vi "STED Control V5.vi"() -> ()   [LabVIEW 2014]
uses:
  Type Defs/Image Acquisition Parameters.ctl
  Laser Controls.ctl
  Detectors.ctl
  Stage Control.ctl
  Focus Control.ctl
  Tools VIs/GrpahTools.ctl
  FPGA-7842R-Reference.ctl
  Scan Parameters.ctl
  Manual Controls V2.ctl
  <vilib>/Utility/miscctls.llb/LVPositionTypeDef.ctl
  <vilib>/Utility/miscctls.llb/LVRectTypeDef.ctl
  Controls/StageStates.ctl
panel:
  in  "Cursor":bool
  in  "Graph Mode":T1(radio)=enum."FullChip"
  in  "Colormap":T2(ring)
  in  "Active Channel":u16(ring) items=["Channel 1"]
  in  "Graph Tools":T3
  in  "Tab Control":T4(tab)
  in  "SLM":bool
  in  "DM":bool
  in  "Timing":bool
  in  "Pixelfly":bool
  in  "Focus Control":T5
  in  "Stage Control":T6={"Halt"=FALSE, "Home"=FALSE, "Down Stage"=FALSE, "Right Stage"=FALSE, "Up Stage"=FALSE, "Left Stage"=FALSE, "X Position"=1.0, "Y Position"=1.0, "Step Size (um)"=enum."1", "Velocity"=enum."Low"} {"Y Position" min=1.0 max=24.0; "X Position" min=1.0 max=24.0}
  out "Channel 6":sgl[][](graph)
  out "Channel 5":sgl[][](graph)
  out "Channel 4":sgl[][](graph)
  out "Channel 3":sgl[][](graph)
  out "Channel 2":sgl[][](graph)
  in  "Detectors":T7
  in  "Laser Controls":T8 {"590 Power (V)" scale=0.0..3.0; "STED Power (V)" scale=0.0..10.0}
  in  "Save File Path":path
  in  "Capture":bool
  out "Channel 1":sgl[][](graph)
  in  "Image Acquisition Parameters":T9={"Scan Type"=enum."Beam Scanning", "Scan Mode"=enum."XY", "Fast Axis Frequency (Hz)"=16110.0, "Image Format"=256, "Line Accumulations"=100, "Frames Per Capture"=1, "Frames Accumulations"=1, "Image Dimension (um)"=[15.0, 15.0], "Number of Z Steps"=1, "Z Steps Size (um)"=1.0, "Pixel Size (nm)"=[58.59375, 58.59375]} {"Z Steps Size (um)" min=0.0; "Number of Z Steps" min=1; "Frames Accumulations" min=1; "Frames Per Capture" min=1; "Line Accumulations" min=1; "Image Format" items=["64 x 64"=64, "128 x 128"=128, "256 x 256"=256, "512 x 512"=512, "1024 x 1024"=1024, "2048 x 2048"=2048]}
  in  "Live":bool
  in  "Exit":bool
  # "XY"
  # "Z"
  # "Length"
  # "Height"
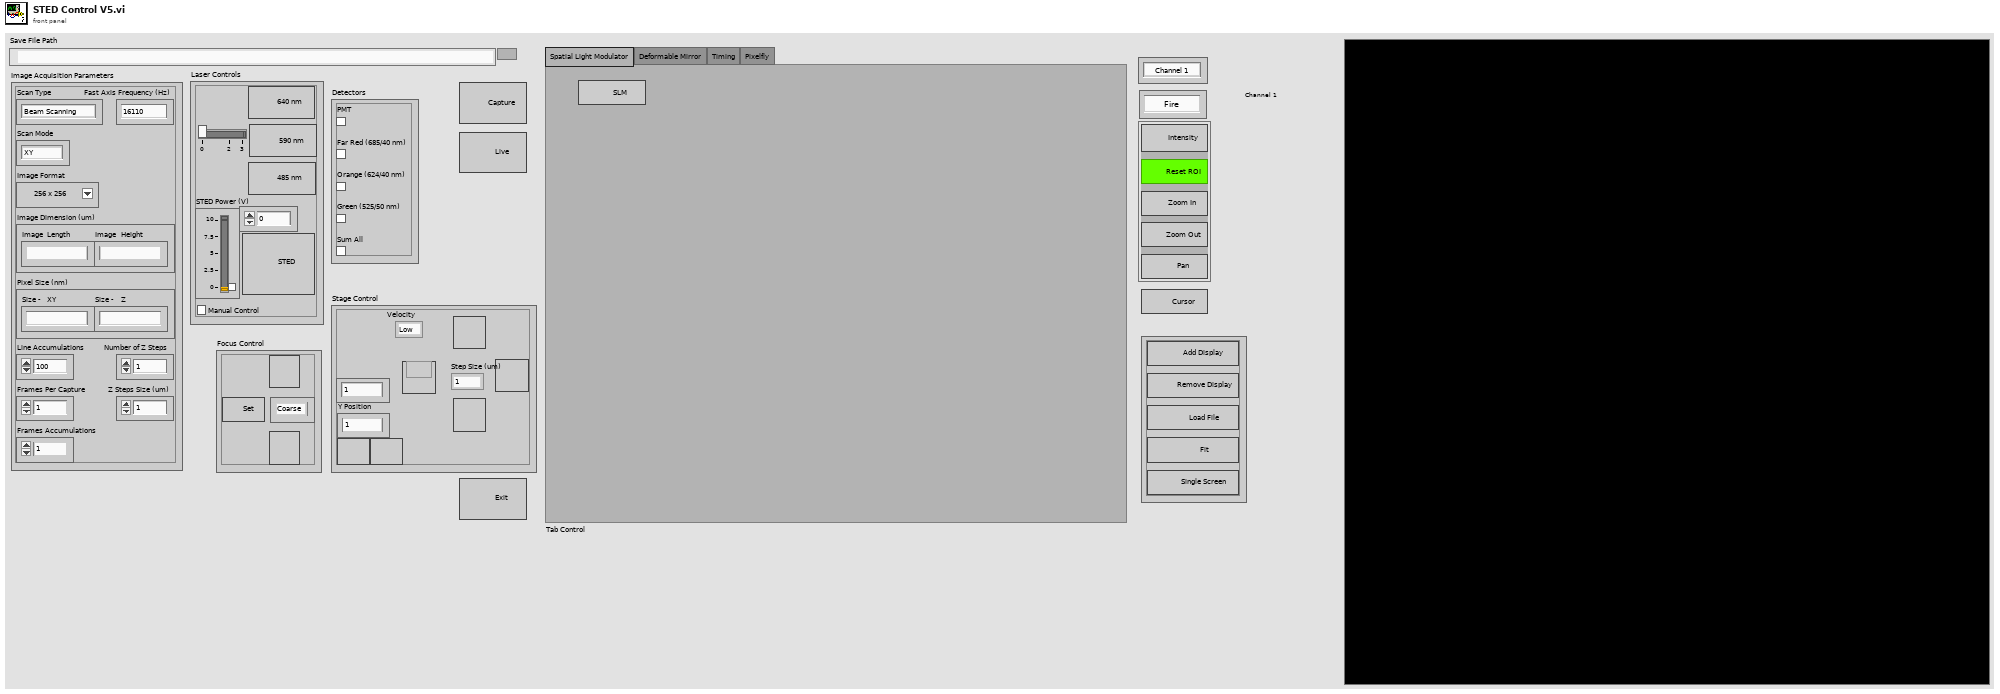
[diagram p1: front panel]
types:
  T1 = enum32{"GetIntensity", "FullChip", "ZoomIn", "ZoomOut", "Pan"}
  T2 = enum16{"Fire", "Gray", "Red", "Green", "Blue", "Cyan", "Magenta", "Yellow", "Red-White", "Green-White", "Blue-White", "Glow"}
  T3 = typedef "GrpahTools.ctl" = cluster{"Add Display":bool, "Remove Display":bool, "Single Screen":bool, "Load File":bool, "Fit":bool}
  T4 = enum32{"Spatial Light Modulator", "Deformable Mirror", "Timing", "Pixelfly"}
  T5 = typedef "Focus Control.ctl" = cluster{"ZoomUp":bool, "ZoomDown":bool, "ZoomStepI16":enum16{"Coarse", "Medium", "Fine"}, "SetZoom":bool}
  T6 = typedef "Stage Control.ctl" = cluster{"Halt":bool, "Home":bool, "Down Stage":bool, "Right Stage":bool, "Up Stage":bool, "Left Stage":bool, "X Position":dbl, "Y Position":dbl, "Step Size (um)":enum16{"1", "2", "5", "10", "15", "20", "50", "100", "500"}, "Velocity":enum16{"Low", "Medium", "High"}}
  T7 = typedef "Detectors.ctl" = cluster{"PMT":bool, "Far Red (685/40 nm)":bool, "Orange (624/40 nm)":bool, "Green (525/50 nm)":bool, "Sum All":bool}
  T8 = typedef "Laser Controls.ctl" = cluster{"STED Power (V)":dbl, "590 Power (V)":dbl, "STED":bool, "640 nm":bool, "590 nm":bool, "485 nm":bool, "Manual Control":bool}
  T9 = typedef "Image Acquisition Parameters.ctl" = cluster{"Scan Type":enum16{"Sample Scanning", "Beam Scanning"}, "Scan Mode":enum16{"XY", "XZ", "YZ", "XYZ"}, "Fast Axis Frequency (Hz)":dbl, "Image Format":u16, "Line Accumulations":u16, "Frames Per Capture":u16, "Frames Accumulations":u16, "Image Dimension (um)":dbl[], "Number of Z Steps":u8, "Z Steps Size (um)":dbl, "Pixel Size (nm)":dbl[]}
  T10 = typedef "Manual Controls V2.ctl" = cluster{"Galvo 1 Position (I16)":i16, "Galvo 2 Position (I16)":i16, "X Axis Voltage (I16)":i16, "Y Axis Voltage (I16)":i16, "Z Axis Voltage (I16)":i16, "Res Mirror Amp (I16)":i16, "Res Mirror Mute":bool}
  T11 = typedef "Scan Parameters.ctl" = cluster{"Fast_Ax_Amp_V":dbl, "Fast_Ax_Off_V":dbl, "Slow_Ax_Amp_V":dbl, "Slow_Ax_Off_V ":dbl, "Slow_Ax_Max_V_VperS":dbl, "Slow_Ax1_Del25ns":i32, "Slow_Ax2_Del25ns":i32, "Stage_X_Off_V":dbl, "Stage_Y_Off_V":dbl, "Stage_Z_Off_V":dbl, "Galvo1_Off_V":dbl, "Galvo2_Off_V":dbl, "Last_Scan_Mode":enum16{"XY", "XZ", "YZ", "XYZ"}, "Current_Scan_Mode":enum16{"XY", "XZ", "YZ", "XYZ"}, "Fly_Back_Lines":u16, "Linear_Ramp_End":u32, "Z_Step_I16":i16, "Z_Start_I16":i16, "Laser_States _U32":u32, "590_Voltage_I16":i16, "775_AOM_Volt_I16":i16, "Blanking OFF":bool, "Unused_Axis_I16":i16}
  T12 = typedef "FPGA-7842R-Reference.ctl" = enum16{"Stage Control", "Laser Control", "Unused Axis I16", "Exit", "Set Res Mirror", "Set Galvo", "Default", "Close FPGA", "Stop Waveforms", "Start Waveforms", "Shutter Control", "Initialize"}
  T13 = enum8{"Enabled", "Disabled", "Disabled and Grayed Out"}
  T14 = typedef "StageStates.ctl" = enum16{"POSITION", "MVR", "MOVE", "HALT", "ONTARGET", "ERROR", "EXIT", "HOME", "ZEROPOS", "NANOPOS", "QUIT", "ANALOG"}
  T15 = typedef "StageStates.ctl" = enum16{"POSITION", "MVR", "MOVE", "HALT", "ONTARGET", "ERROR", "EXIT", "HOME", "ZEROPOS", "NANOPOS", "QUIT", "SERVO", "JOYSTICK", "ANALOG"}
  T16 = typedef "LVPositionTypeDef.ctl" = cluster{"Left":i32, "Top":i32}
  T17 = typedef "LVRectTypeDef.ctl" = cluster{"Left":i16, "Top":i16, "Right":i16, "Bottom":i16}
  T18 = enum32{"Invalid", "Standard", "Closed", "Hidden", "Minimized", "Maximized"}
  T19 = cluster{"Halt":bool, "Home":bool, "Down Stage":bool, "Right Stage":bool, "Up Stage":bool, "Left Stage":bool, "X Position":bool, "Y Position":bool, "Step Size (um)":bool, "Velocity":bool}
  T20 = enum16{"1", "2", "5", "10", "15", "20", "50", "100", "500"}
  T21 = typedef "Scanning Conversions.ctl" = cluster{"Stage X Axis (Volts/um)":dbl, "Stage Y Axis (Volts/um)":dbl, "Stage Z Axis (Volts/um)":dbl}
  T22 = cluster{"Scan Type":bool, "Scan Mode":bool, "Fast Axis Frequency (Hz)":bool, "Image Format":bool, "Line Accumulations":bool, "Frames Per Capture":bool, "Frames Accumulations":bool, "Image Dimension (um)":bool[], "Number of Z Steps":bool, "Z Steps Size (um)":bool, "Pixel Size (nm)":bool[]}
  T23 = typedef "LVAllMonitorsDisplayTypeDef.ctl" = cluster{"Bounds":cluster{"Left":i16, "Top":i16, "Right":i16, "Bottom":i16}, "Depth":i16}[]
  T24 = cluster{"Bounds":cluster{"Left":i16, "Top":i16, "Right":i16, "Bottom":i16}, "Depth":i16}
  T25 = typedef "IMAQ Image.ctl" = refnum<image>
  T26 = typedef "Waveform Data.ctl" = cluster{"Waveform Scan Parameters":cluster{"Scanning Mode":u8, "Fast Axis WF Length (Elements)":i32, "Fast Axis Sample Period (Ticks)":u32, "Slow Axis 1 WF Length (Elements)":i32, "Slow Axis 1 Sample Period (Ticks)":u32, "Slow Axis 1 Delay (25 ns) Steps":i32, "Slow Axis 2 WFLength (Elements)":i32, "Slow Axis 2 Sample Period (Ticks)":u32, "Slow Axis 2 Delay (25 ns) Steps":i32}, "Fast Axis Waveform":dbl[], "Slow Axis 1 Waveform":dbl[], "Slow Axis 2 Waveform":dbl[]}
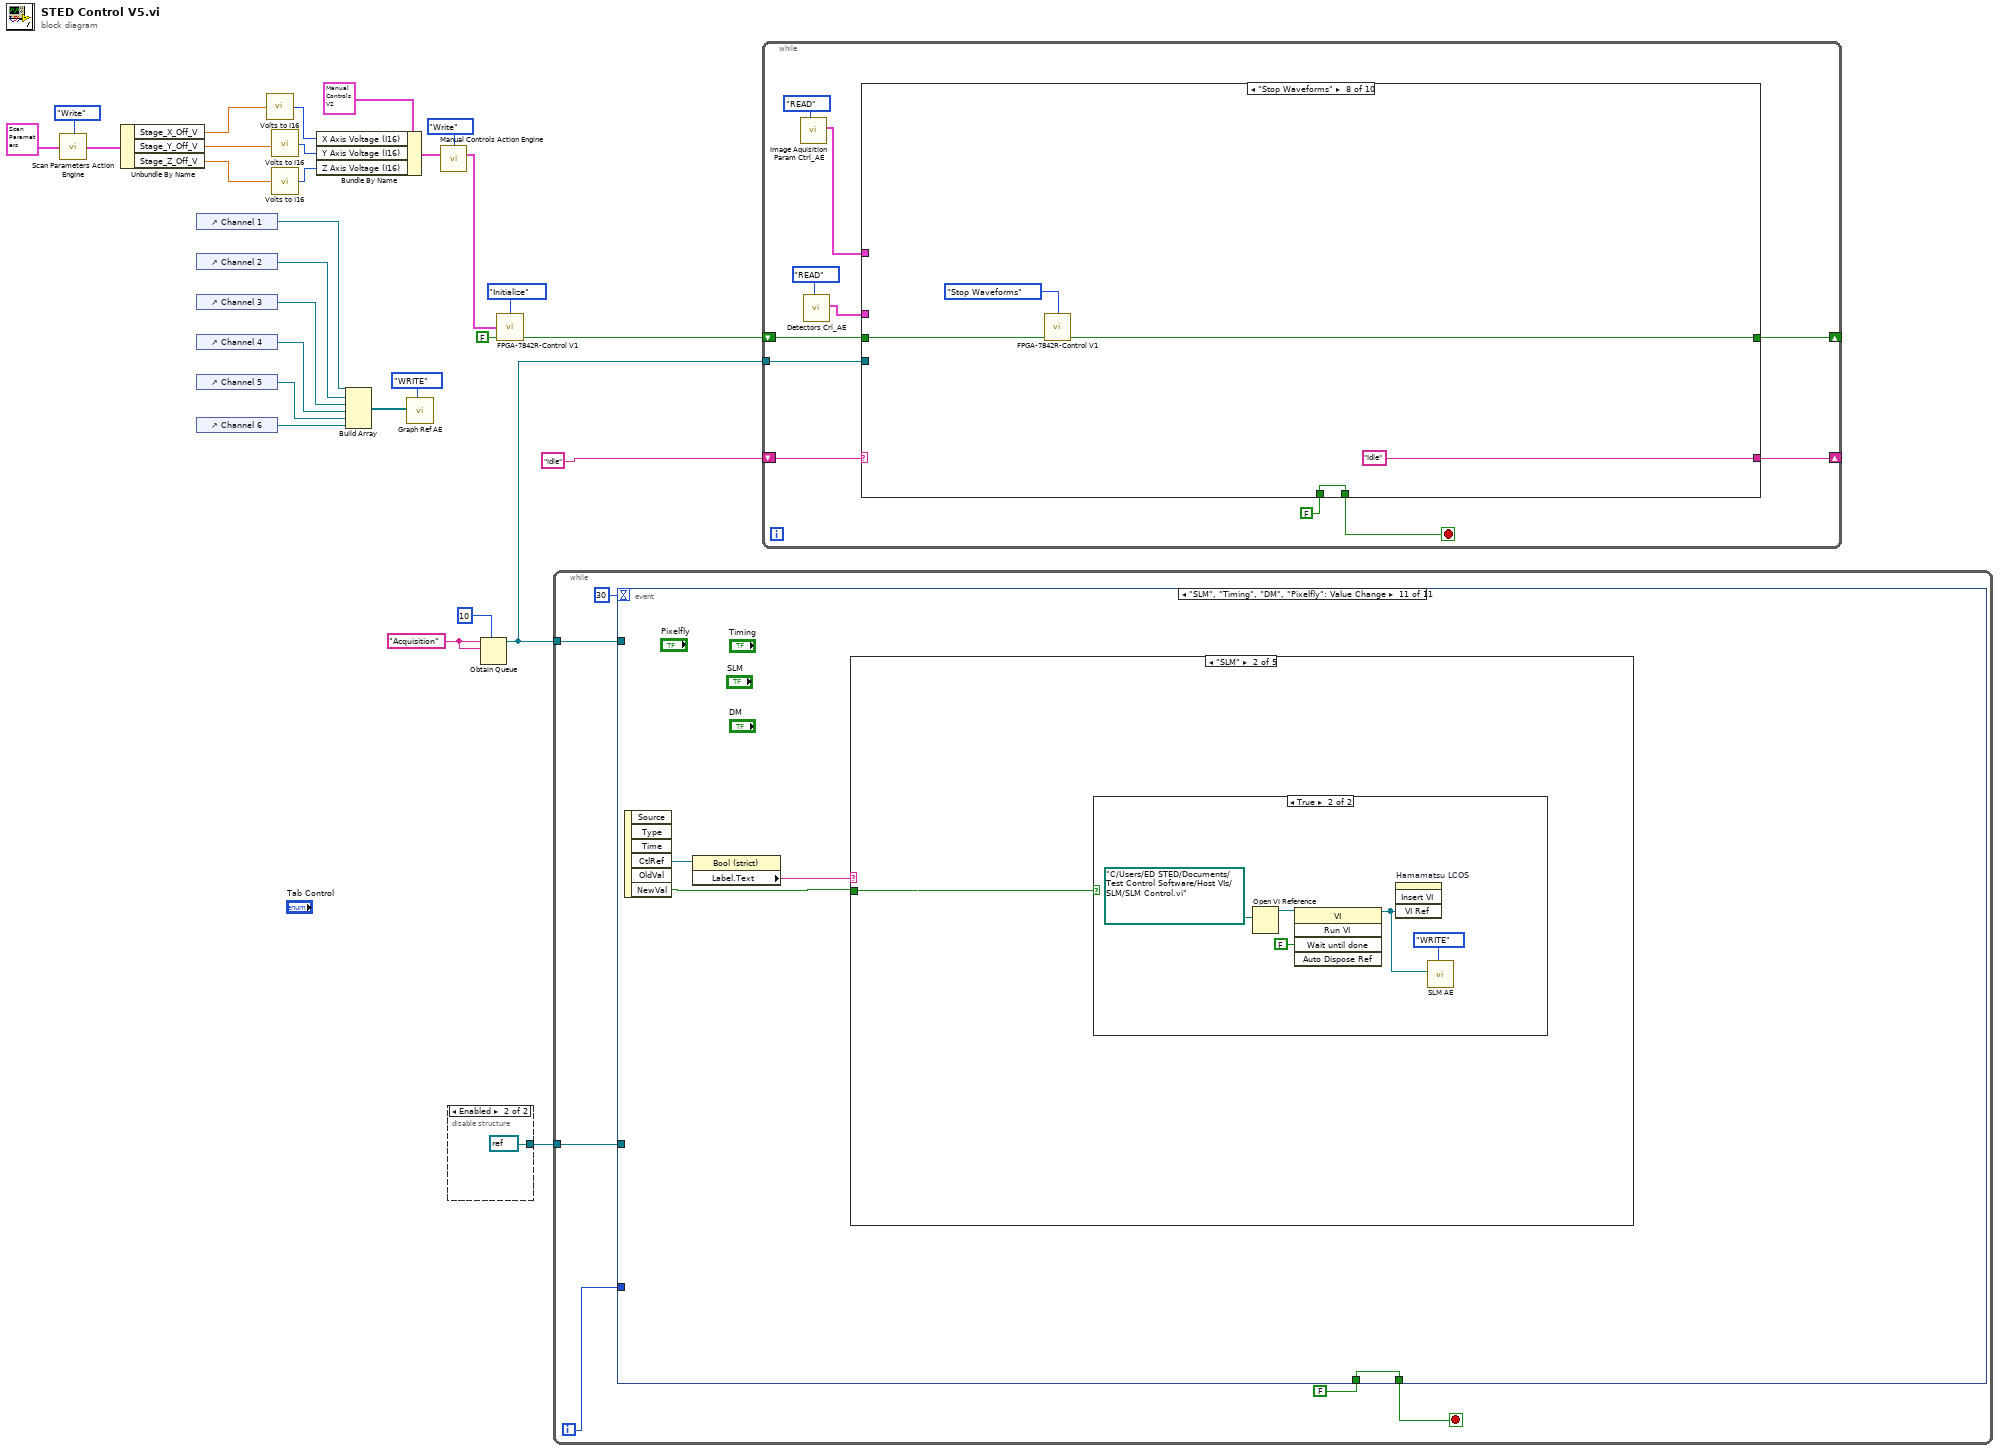
[diagram p0: block diagram]
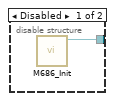
[diagram p2: hidden frame]
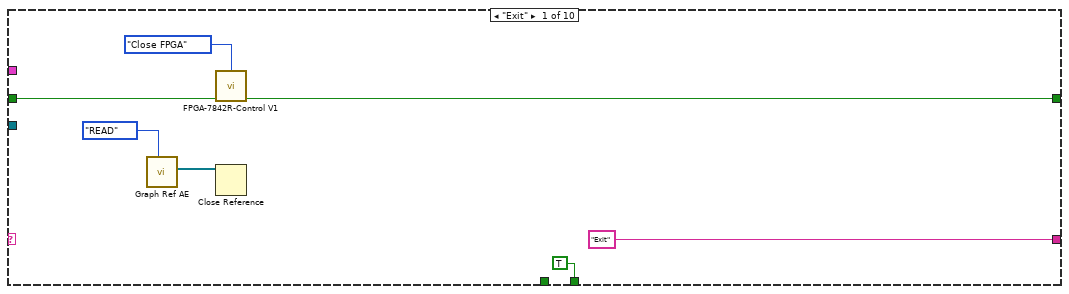
[diagram p3: hidden frame]
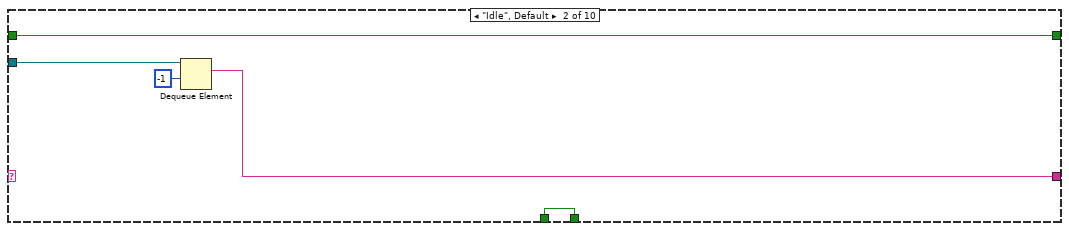
[diagram p4: hidden frame]
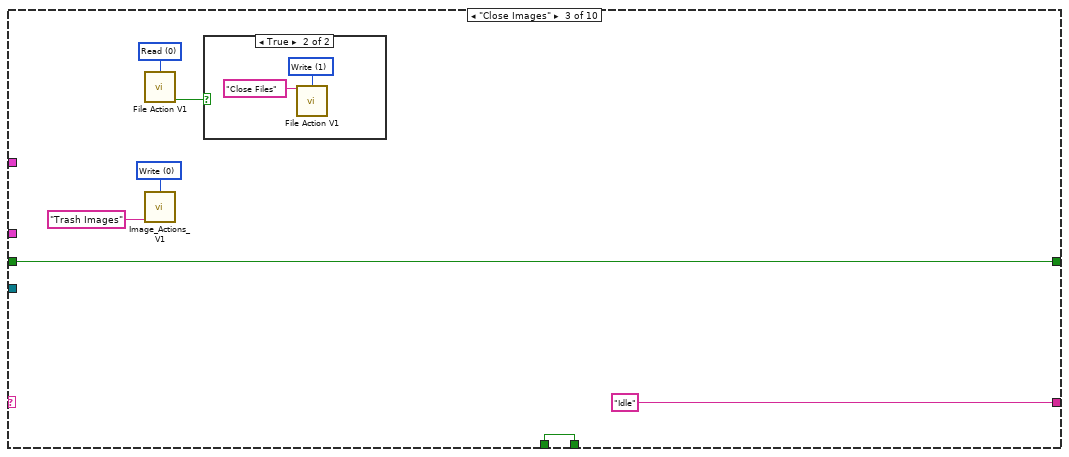
[diagram p5: hidden frame]
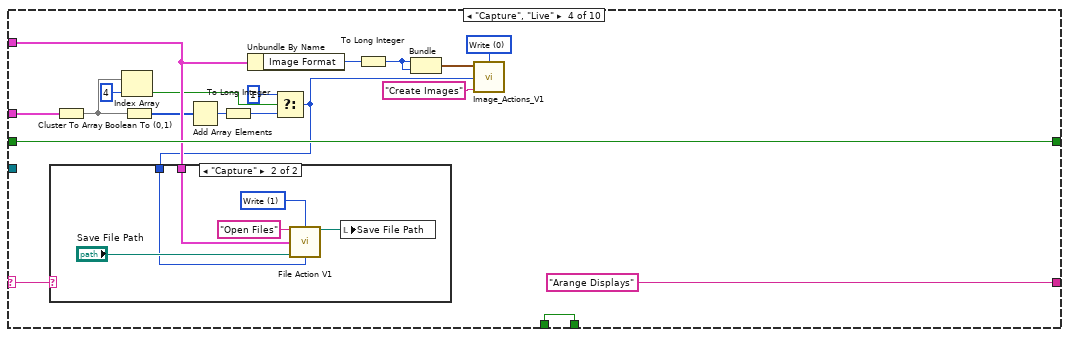
[diagram p7: hidden frame]
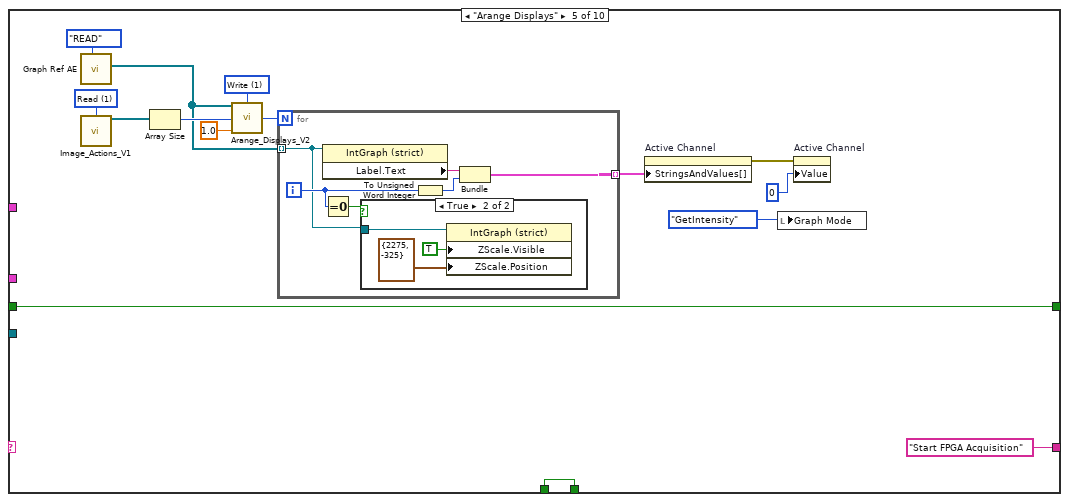
[diagram p9: hidden frame]
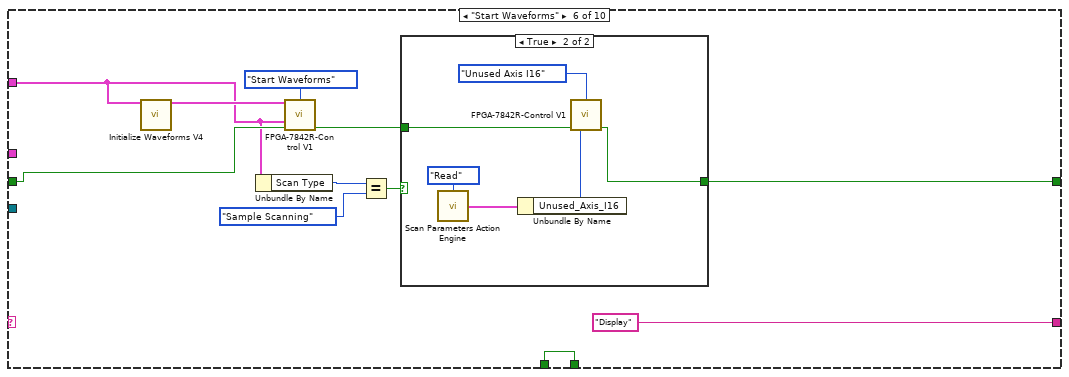
[diagram p11: hidden frame]
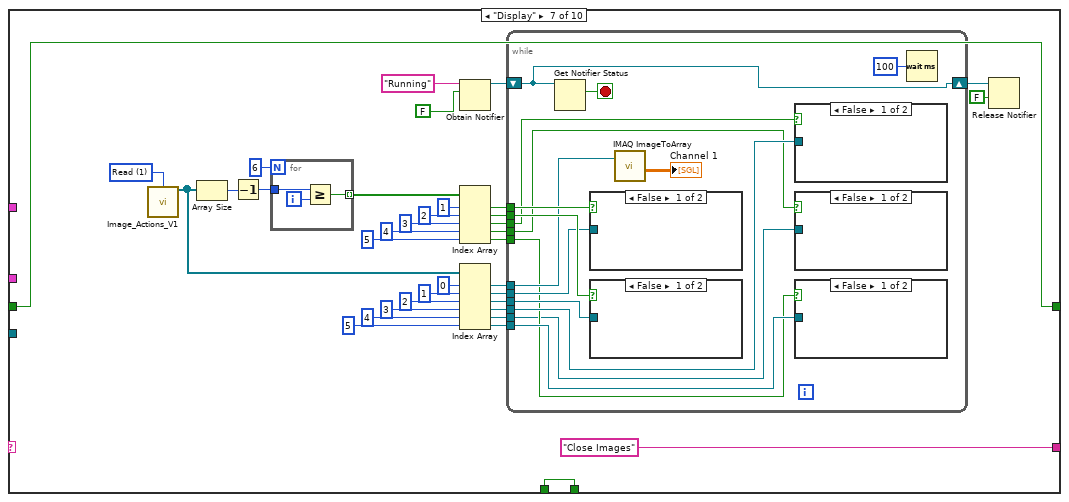
[diagram p13: hidden frame]
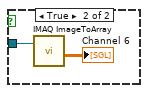
[diagram p14: hidden frame]
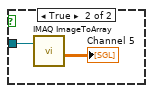
[diagram p15: hidden frame]
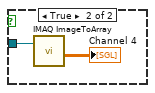
[diagram p16: hidden frame]
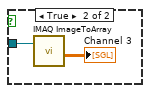
[diagram p17: hidden frame]
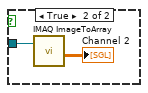
[diagram p18: hidden frame]
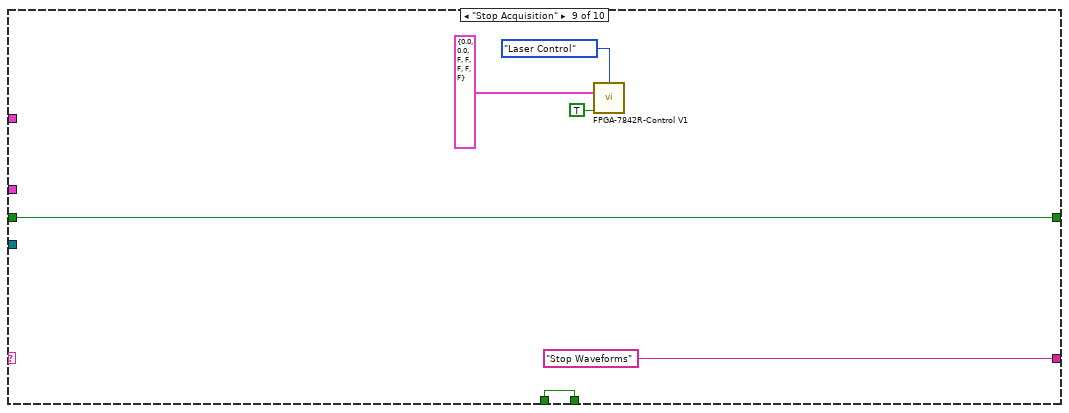
[diagram p19: hidden frame]
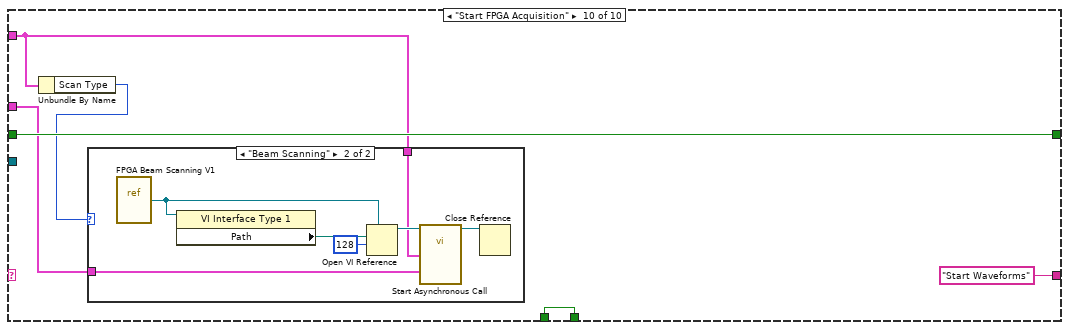
[diagram p20: hidden frame]
diagram:
  w28 = "Acquisition" ("name (unnamed)")
  n1 = call "Scan Parameters Action Engine.vi"("Action"=enum16{"Read", "Write"}."Write", "Scan Parameters IN"=T11 {"Fast_Ax_Amp_V"=0.0, "Fast_Ax_Off_V"=0.0, "Slow_Ax_Amp_V"=0.0, "Slow_Ax_Off_V "=0.0, "Slow_Ax_Max_V_VperS"=0.0, "Slow_Ax1_Del25ns"=0, "Slow_Ax2_Del25ns"=0, "Stage_X_Off_V"=5.0, "Stage_Y_Off_V"=5.0, "Stage_Z_Off_V"=5.0, "Galvo1_Off_V"=0.0, "Galvo2_Off_V"=0.0, "Last_Scan_Mode"=enum."XY", "Current_Scan_Mode"=enum."XY", "Fly_Back_Lines"=0, "Linear_Ramp_End"=0, "Z_Step_I16"=0, "Z_Start_I16"=0, "Laser_States _U32"=0, "590_Voltage_I16"=0, "775_AOM_Volt_I16"=0, "Blanking OFF"=FALSE, "Unused_Axis_I16"=16384}) -> ("Scan Parameters OUT"=w11:T11)  [unwired: 13 in]
  n2 = Unbundle By Name(w11) -> ("Stage_X_Off_V"=w7:dbl, "Stage_Y_Off_V"=w6:dbl, "Stage_Z_Off_V"=w5:dbl)
  n3 = control-ref of="Channel 1"() -> (w3:refnum<vi>)
  n4 = control-ref of="Channel 2"() -> (w20:refnum<vi>)
  n5 = control-ref of="Channel 3"() -> (w4:refnum<vi>)
  n6 = control-ref of="Channel 4"() -> (w19:refnum<vi>)
  n7 = control-ref of="Channel 5"() -> (w18:refnum<vi>)
  n8 = control-ref of="Channel 6"() -> (w17:refnum<vi>)
  n9 = call "Volts to I16.vi"("Voltage (V)"=w7) -> ("I16"=w8:i16)  [unwired: 13 in, 1 out]
  n10 = call "Volts to I16.vi"("Voltage (V)"=w6) -> ("I16"=w9:i16)  [unwired: 13 in, 1 out]
  n11 = call "Volts to I16.vi"("Voltage (V)"=w5) -> ("I16"=w10:i16)  [unwired: 13 in, 1 out]
  n12 = Bundle By Name(cluster=T10 {"Galvo 1 Position (I16)"=-280, "Galvo 2 Position (I16)"=0, "X Axis Voltage (I16)"=16384, "Y Axis Voltage (I16)"=16384, "Z Axis Voltage (I16)"=16384, "Res Mirror Amp (I16)"=0, "Res Mirror Mute"=FALSE} ("Manual Controls"), "X Axis Voltage (I16)"=w8, "Y Axis Voltage (I16)"=w9, "Z Axis Voltage (I16)"=w10) -> (w12:T10)
  n13 = Build Array(w3, w20, w4, w19, w18, w17) -> (w1:refnum<vi>[])
  n14 = call "Graph Ref AE.vi"("Action"=enum16{"READ", "WRITE"}."WRITE", "Graph Ref In"=w1) -> ()  [unwired: 9 in, 1 out]
  n15 = call "Manual Controls Action Engine.vi"("Action"=enum16{"Read", "Write"}."Write", "Manual Controls In"=w12) -> ("Manual Controls Out"=w14:T10)  [unwired: 13 in]
  n16 = disable-structure shown="Enabled" {
    disable-tunnel: [w30 refnum<visa-resource-name> refnum ("VISA Refnum out")] -> w16
    frame Disabled {
      n17 = call "M686_Init.vi"() -> ("VISA Refnum out"=w30:refnum<visa-resource-name>)  [unwired: 9 in, 2 out]
    }
    frame Enabled {
    }
  }
  n18 = Obtain Queue(max queue size (-1, unlimited)=10, name (unnamed)=w28, element data type=w28) -> (queue out=w26:refnum<queue>)  [unwired: 2 in, 2 out]
  n19 = call "FPGA-7842R-Control V1.vi"("Action"=FPGA-7842R-Reference."Initialize", "Manual Controls"=w14, "Initialize"=FALSE) -> ("Initalized"=w23:bool)  [unwired: 11 in, 1 out]
  n20 = while {
    tunnel: w26 -> [w35]
    tunnel: w16 -> [w33]
    i -> [w32]
    stop <- w37 stop-if-true
    n21 = event shown="[10] \"SLM\", \"Timing\", \"DM\", \"Pixelfly\": Value Change" {
      selector: _ -> [_ _ _ _ _ _ _ _ _ _ _]
      dyn-events: _ -> [_ _ _ _ _ _ _ _ _ _ _]
      timeout: 30 -> [_ _ _ _ _ _ _ _ _ _ _]
      tunnel: [w54 w88 w107 w117 w305 w332 w369 w408 w523 w601 w702] -> w37
      tunnel: FALSE -> [_ w88 w107 w117 w305 w332 w369 w408 w523 w601 w702]
      tunnel: w35 -> [w53 w87 w101 _ _ _ _ _ _ _ _]
      tunnel: w33 -> [w50 _ _ w116 _ _ _ _ _ _ _]
      tunnel: w32 -> [_ _ w99 _ _ _ _ _ _ _ _]
      event "Exit": Value Change {
        n22 = event-data() -> ("CtlRef"=w52:refnum<vi>, "NewVal"=w54:bool)  [unwired: 1 in, 4 out]
        n23 = disable-structure shown="Disabled" {
          disable-tunnel: w50 -> [w55 _]
          frame Disabled {
            n24 = call "M686_Quit.vi"("VISA Refnum in"=w55) -> ()  [unwired: 11 in]
          }
          frame Enabled {
          }
        }
        n25 = call "SLM AE.vi"("Action"=enum16{"READ", "WRITE"}."READ") -> ("SLM Ref Out"=w47:refnum<vi>)  [unwired: 10 in]
        n26 = Not A Number/Path/Refnum?(number/path/refnum=w47) -> (NaN/Path/Refnum?=w48:bool)
        n27 = case shown="False" w48 {
          tunnel: w47 -> [w71 _]
          frame False {
            n28 = To Variant(anything=TRUE) -> (Variant=w72:variant)
            n29 = invoke class="VI" method="Ctrl Val.Set"(reference=w71, "Control Name"="Exit", "Value"=w72) -> (reference out=w75:refnum<vi>)  [unwired: 2 in, 4 out]
            n30 = Close Reference(reference=w75) -> ()  [unwired: 1 in, 1 out]
          }
          frame True {
          }
        }
        n31 = property class="Bool"(reference=w52) -> ("Label.Text"=w51:string)  [unwired: 1 in, 2 out]
        n32 = Enqueue Element(queue=w53, element=w51) -> ()  [unwired: 2 in, 3 out]
        n33 = call "GateDelay AE.vi"("Action"=enum16{"READ", "WRITE"}."READ") -> ("Gate Delay Ref Out"=w46:refnum<vi>)  [unwired: 10 in]
        n34 = call "DM_Ref_AE.vi"("Action"=enum16{"READ", "WRITE"}."READ") -> ("DM Ref Out"=w41:refnum<vi>)  [unwired: 10 in]
        n35 = Not A Number/Path/Refnum?(number/path/refnum=w46) -> (NaN/Path/Refnum?=w45:bool)
        n36 = case shown="False" w45 {
          tunnel: w46 -> [w66 _]
          frame False {
            n37 = To Variant(anything=TRUE) -> (Variant=w67:variant)
            n38 = invoke class="VI" method="Ctrl Val.Set"(reference=w66, "Control Name"="Exit", "Value"=w67) -> (reference out=w70:refnum<vi>)  [unwired: 2 in, 4 out]
            n39 = Close Reference(reference=w70) -> ()  [unwired: 1 in, 1 out]
          }
          frame True {
          }
        }
        n40 = Not A Number/Path/Refnum?(number/path/refnum=w41) -> (NaN/Path/Refnum?=w43:bool)
        n41 = case shown="False" w43 {
          tunnel: w41 -> [w61 _]
          frame False {
            n42 = To Variant(anything=TRUE) -> (Variant=w62:variant)
            n43 = invoke class="VI" method="Ctrl Val.Set"(reference=w61, "Control Name"="Exit", "Value"=w62) -> (reference out=w65:refnum<vi>)  [unwired: 2 in, 4 out]
            n44 = Close Reference(reference=w65) -> ()  [unwired: 1 in, 1 out]
          }
          frame True {
          }
        }
        n45 = call "Pixelfly AE.vi"("Action"=enum16{"READ", "WRITE"}."READ") -> ("Gate Delay Ref Out"=w38:refnum<vi>)  [unwired: 10 in]
        n46 = Not A Number/Path/Refnum?(number/path/refnum=w38) -> (NaN/Path/Refnum?=w39:bool)
        n47 = case shown="False" w39 {
          tunnel: w38 -> [w56 _]
          frame False {
            n48 = To Variant(anything=TRUE) -> (Variant=w57:variant)
            n49 = invoke class="VI" method="Ctrl Val.Set"(reference=w56, "Control Name"="Exit", "Value"=w57) -> (reference out=w60:refnum<vi>)  [unwired: 2 in, 4 out]
            n50 = Close Reference(reference=w60) -> ()  [unwired: 1 in, 1 out]
          }
          frame True {
          }
        }
      }
      event "Live", "Capture": Value Change {
        n51 = event-data() -> ("CtlRef"=w86:refnum<vi>, "NewVal"=w76:bool)  [unwired: 1 in]
        n52 = property class="Bool (strict)"(reference=w86) -> ("Label.Text"=w77:string)  [unwired: 1 in, 2 out]
        n53 = Obtain Notifier(name (unnamed)="Running", notification data type=TRUE) -> (notifier out=w83:refnum<notifier>)  [unwired: 2 in, 2 out]
        n54 = Not(x=w76) -> (.not. x?=w81:bool)
        n55 = Send Notification(notification=w81, notifier=w83) -> (notifier out=w79:refnum<notifier>)  [unwired: 1 in, 1 out]
        n56 = case shown="\"Live\"" w77 {
          tunnel: w76 -> [_ w90 w94]
          frame "False", Default {
          }
          frame "Live" {
            n57 = case shown="True" w90 {
              tunnel: [T13."Enabled" ("Disabled") T13."Disabled and Grayed Out" ("Disabled")] -> w89
              frame False {
              }
              frame True {
              }
            }
            n58 = property on="Capture" class="Bool (strict)"("DisabledEnum"=w89) -> ()  [unwired: 2 in, 2 out]
            n59 = property on="Exit" class="Bool"("DisabledEnum"=w89) -> ()  [unwired: 2 in, 2 out]
          }
          frame "Capture" {
            n60 = case shown="True" w94 {
              tunnel: [T13."Enabled" ("Disabled") T13."Disabled and Grayed Out" ("Disabled")] -> w93
              frame False {
              }
              frame True {
              }
            }
            n61 = property on="Live" class="Bool (strict)"("DisabledEnum"=w93) -> ()  [unwired: 2 in, 2 out]
            n62 = property on="Exit" class="Bool"("DisabledEnum"=w93) -> ()  [unwired: 2 in, 2 out]
          }
        }
        n63 = Release Notifier(notifier=w79, force destroy? (F)=FALSE) -> ()  [unwired: 1 in, 3 out]
        n64 = Select(t=w77, s=w76, f="Stop Acquisition") -> (s? t:f=w80:string)
        n65 = Enqueue Element(queue=w87, element=w80) -> ()  [unwired: 2 in, 3 out]
      }
      event Timeout {
        n66 = event-data() -> ()  [unwired: 1 in, 3 out]
        n67 = Equal To 0?(x=w99) -> (x = 0?=w98:bool)
        n68 = Obtain Notifier(name (unnamed)="Running", notification data type=TRUE) -> (notifier out=w105:refnum<notifier>)  [unwired: 2 in, 2 out]
        n69 = Get Notifier Status(notifier=w105) -> (notifier out=w97:refnum<notifier>, current notification=w103:bool)  [unwired: 1 in, 3 out]
        n70 = case shown="False" w98 {
          frame False {
            n71 = call "Image Aquisition Param Ctrl_AE.vi"("Action"=enum16{"READ", "WRITE"}."READ") -> ("Image Acquisition Parameters Out"=w109:T9)  [unwired: 10 in]
            n72 = local write "Image Acquisition Parameters"(w109) -> ()
          }
          frame True {
            n73 = local read "Image Acquisition Parameters"() -> (w110:T9)
            n74 = call "Image Aquisition Param Ctrl_AE.vi"("Action"=enum16{"READ", "WRITE"}."WRITE", "Image Acquisition Parameters In"=w110) -> ()  [unwired: 9 in, 1 out]
          }
        }
        n75 = Release Notifier(notifier=w97) -> ()  [unwired: 2 in, 3 out]
        n76 = local read "Capture"() -> (w102:bool)
        n77 = And(x=w103, y=w102) -> (x .and. y?=w100:bool)
        n78 = case shown="True" w100 {
          tunnel: w101 -> [_ w114]
          frame False {
          }
          frame True {
            n79 = local write "Capture"(FALSE ("Capture")) -> ()
            n80 = Enqueue Element(queue=w114, element="Stop Acquisition" ("f")) -> ()  [unwired: 2 in, 3 out]
            n81 = property on="Live" class="Bool (strict)"("DisabledEnum"=T13."Enabled" ("Disabled")) -> ()  [unwired: 2 in, 2 out]
          }
        }
      }
      event Value Change {
        n82 = event-data() -> ("OldVal"=w119:T6, "NewVal"=w118:T6)  [unwired: 1 in, 4 out]
        n83 = disable-structure shown="Disabled" {
          disable-tunnel: w119 -> [w139 _]
          disable-tunnel: w118 -> [w138 _]
          disable-tunnel: w116 -> [w124 _]
          frame Disabled {
            n84 = property on="Stage Control" class="Clust"() -> ("Controls[]"=w126:refnum<vi>[])  [unwired: 2 in, 2 out]
            n85 = Not Equal?(x=w139, y=w138) -> (x != y?=w125:T19)
            n86 = Unbundle By Name(w138) -> ("Mode"=w132:enum32{"Joystick", "Coarse", "Fine"}, "Step Size (um)"=w131:T20, "Velocity"=w129:enum16{"Low", "Medium", "High"})
            n87 = Cluster To Array(cluster=w125) -> (array=w134:bool[])
            n88 = for {
              tunnel: w126 -> [w298] mode=indexing
              tunnel: w134 -> [w299] mode=indexing
              tunnel: [w298] -> w135
              stop <- w299 stop-if-true
            }
            n89 = Format Into String(w129) -> (resulting string=w128:string)  [unwired: 3 in, 1 out]
            n90 = Format Into String(w131) -> (resulting string=w133:string)  [unwired: 3 in, 1 out]
            n91 = case shown="\"Medium\", Default" w128 {
              tunnel: [0.5 1.0 0.1] -> w127
              frame "Medium", Default {
              }
              frame "High" {
              }
              frame "Low" {
              }
            }
            n92 = property class="Ctl"(reference=w135) -> ("ClassName"=w136:string, "Label.Text"=w137:string)  [unwired: 1 in, 2 out]
            n93 = control-ref of="Halt"() -> (w122:refnum<vi>)
            n94 = Fract/Exp String To Number(string=w133) -> (number=w130:dbl)  [unwired: 3 in, 1 out]
            n95 = case shown="\"Joystick\"" w132 {
              tunnel: w124 -> [w148 w161 w232 w243]
              tunnel: w136 -> [_ w160 _ w242]
              tunnel: w137 -> [_ w159 _ w241]
              tunnel: [w147 w158 w231 w240] -> w123
              tunnel: w122 -> [w146 w157 w230 w238]
              tunnel: w130 -> [_ w156 _ w239]
              tunnel: w127 -> [w145 w155 _ _]
              frame "Joystick" {
                w143 = TRUE
                n96 = Build Array(w143, w143) -> (w142:bool[])
                n97 = call "M686.vi"("Velocity"=w145, "Abort"=w146, "Axis"=w142, "Action"=StageStates."JOYSTICK", "VISA In"=w148) -> ("VISA Out"=w141:refnum<visa-resource-name>)  [unwired: 3 in, 3 out]
                n98 = call "M686.vi"("Abort"=w146, "Action"=StageStates."POSITION", "VISA In"=w141) -> ("Position Out"=w147:dbl[])  [unwired: 5 in, 3 out]
              }
              frame "Coarse" {
                w153 = FALSE
                n99 = Build Array(w153, w153) -> (w152:bool[])
                n100 = call "M686.vi"("Abort"=w157, "Axis"=w152, "Action"=StageStates."JOYSTICK", "VISA In"=w161) -> ("VISA Out"=w151:refnum<visa-resource-name>)  [unwired: 4 in, 3 out]
                n101 = Divide(x=w156, y=1000.0) -> (x/y=w150:dbl)
                n102 = case shown="\"Boolean\"" w160 {
                  tunnel: w159 -> [_ w171]
                  tunnel: w151 -> [w165 w170]
                  tunnel: w150 -> [_ w169]
                  tunnel: w157 -> [w162 w168]
                  tunnel: [w164 w167] -> w158
                  tunnel: w155 -> [_ w166]
                  frame Default {
                    n103 = call "M686.vi"("Abort"=w162, "Action"=StageStates."POSITION", "VISA In"=w165) -> ("Position Out"=w164:dbl[])  [unwired: 5 in, 3 out]
                  }
                  frame "Boolean" {
                    n104 = case shown="\"Right Stage\"" w171 {
                      tunnel: w170 -> [_ w176 w186 w194 w207 w217 w228]
                      tunnel: w169 -> [_ _ _ w193 w206 w208 w227]
                      tunnel: w168 -> [_ w174 w185 w195 w205 w216 w226]
                      tunnel: [dbl[] [] ("Position Out") w173 w184 w196 w204 w215 w225] -> w167
                      tunnel: w166 -> [_ _ _ w192 w203 w214 w224]
                      frame Default {
                      }
                      frame "Home" {
                        w178 = TRUE
                        n105 = Build Array(w178, w178) -> (w179:bool[])
                        n106 = call "M686.vi"("Velocity"=1.0, "Abort"=w174, "Axis"=w179, "Action"=StageStates."HOME", "VISA In"=w176) -> ("Position Out"=w173:dbl[])  [unwired: 3 in, 3 out]
                      }
                      frame "Halt" {
                        w182 = TRUE
                        n107 = Build Array(w182, w182) -> (w183:bool[])
                        n108 = call "M686.vi"("Velocity"=1.0, "Abort"=w185, "Axis"=w183, "Action"=StageStates."HALT", "VISA In"=w186) -> ("Position Out"=w184:dbl[])  [unwired: 3 in, 3 out]
                      }
                      frame "Up Stage" {
                        n109 = Build Array(w193, w193) -> (w190:dbl[])
                        n110 = Build Array(FALSE, TRUE) -> (w187:bool[])
                        n111 = call "M686.vi"("Velocity"=w192, "Abort"=w195, "Axis"=w187, "Positions"=w190, "Action"=StageStates."MVR", "VISA In"=w194) -> ("Position Out"=w196:dbl[])  [unwired: 2 in, 3 out]
                      }
                      frame "Down Stage" {
                        n112 = Negate(x=w206) -> (-x=w197:dbl)
                        n113 = Build Array(w197, w197) -> (w201:dbl[])
                        n114 = Build Array(FALSE, TRUE) -> (w198:bool[])
                        n115 = call "M686.vi"("Velocity"=w203, "Abort"=w205, "Axis"=w198, "Positions"=w201, "Action"=StageStates."MVR", "VISA In"=w207) -> ("Position Out"=w204:dbl[])  [unwired: 2 in, 3 out]
                      }
                      frame "Left Stage" {
                        n116 = Build Array(w208, w208) -> (w212:dbl[])
                        n117 = Build Array(TRUE, FALSE) -> (w209:bool[])
                        n118 = call "M686.vi"("Velocity"=w214, "Abort"=w216, "Axis"=w209, "Positions"=w212, "Action"=StageStates."MVR", "VISA In"=w217) -> ("Position Out"=w215:dbl[])  [unwired: 2 in, 3 out]
                      }
                      frame "Right Stage" {
                        n119 = Negate(x=w227) -> (-x=w218:dbl)
                        n120 = Build Array(w218, w218) -> (w222:dbl[])
                        n121 = Build Array(TRUE, FALSE) -> (w219:bool[])
                        n122 = call "M686.vi"("Velocity"=w224, "Abort"=w226, "Axis"=w219, "Positions"=w222, "Action"=StageStates."MVR", "VISA In"=w228) -> ("Position Out"=w225:dbl[])  [unwired: 2 in, 3 out]
                      }
                    }
                  }
                }
              }
              frame Default {
                n123 = call "M686.vi"("Abort"=w230, "Action"=StageStates."POSITION", "VISA In"=w232) -> ("Position Out"=w231:dbl[])  [unwired: 5 in, 3 out]
              }
              frame "Fine" {
                w236 = FALSE
                n124 = case shown="\"Boolean\"" w242 {
                  tunnel: w241 -> [_ w253]
                  tunnel: w239 -> [_ w252]
                  frame "False", Default {
                  }
                  frame "Boolean" {
                    n125 = call "Manual Controls Action Engine.vi"("Action"=enum16{"Read", "Write"}."Read") -> ("Manual Controls Out"=w250:T10)  [unwired: 14 in]
                    n126 = call "Scanning Volts to Microns.vi"() -> ("Scanning Conversions OUT"=w251:T21)
                    n127 = case shown="Default" w253 {
                      tunnel: w252 -> [_ w262 _ w275 w284 w293]
                      tunnel: w251 -> [_ w263 _ w276 w285 w294]
                      tunnel: w250 -> [w254 w261 w267 w274 w283 w292]
                      tunnel: [w254 w260 w266 w273 w282 w291] -> w248
                      frame Default {
                      }
                      frame "Up Stage" {
                        n128 = Unbundle By Name(w263) -> ("Stage Y Axis (Volts/um)"=w259:dbl)
                        n129 = Unbundle By Name(w261) -> ("Y Axis Voltage (I16)"=w258:i16)
                        n130 = Multiply(x=w262, y=w259) -> (x*y=w256:dbl)
                        n131 = call "Volts to I16.vi"("Voltage (V)"=w256) -> ("I16"=w255:i16)  [unwired: 13 in, 1 out]
                        n132 = Subtract(x=w258, y=w255) -> (x-y=w257:i16)
                        n133 = Bundle By Name(cluster=w261, "Y Axis Voltage (I16)"=w257) -> (w260:T10)
                      }
                      frame "Home" {
                        n134 = call "Volts to I16.vi"("Voltage (V)"=5.0 ("Stage Y Axis Offset (V)")) -> ("I16"=w264:i16)  [unwired: 13 in, 1 out]
                        n135 = Bundle By Name(cluster=w267, "X Axis Voltage (I16)"=w264, "Y Axis Voltage (I16)"=w264) -> (w266:T10)
                      }
                      frame "Down Stage" {
                        n136 = Unbundle By Name(w274) -> ("Y Axis Voltage (I16)"=w271:i16)
                        n137 = Unbundle By Name(w276) -> ("Stage Y Axis (Volts/um)"=w272:dbl)
                        n138 = Multiply(x=w275, y=w272) -> (x*y=w269:dbl)
                        n139 = call "Volts to I16.vi"("Voltage (V)"=w269) -> ("I16"=w268:i16)  [unwired: 13 in, 1 out]
                        n140 = Add(x=w271, y=w268) -> (x+y=w270:i16)
                        n141 = Bundle By Name(cluster=w274, "Y Axis Voltage (I16)"=w270) -> (w273:T10)
                      }
                      frame "Left Stage" {
                        n142 = Unbundle By Name(w285) -> ("Stage X Axis (Volts/um)"=w281:dbl)
                        n143 = Unbundle By Name(w283) -> ("X Axis Voltage (I16)"=w280:i16)
                        n144 = Multiply(x=w284, y=w281) -> (x*y=w278:dbl)
                        n145 = call "Volts to I16.vi"("Voltage (V)"=w278) -> ("I16"=w277:i16)  [unwired: 13 in, 1 out]
                        n146 = Subtract(x=w280, y=w277) -> (x-y=w279:i16)
                        n147 = Bundle By Name(cluster=w283, "X Axis Voltage (I16)"=w279) -> (w282:T10)
                      }
                      frame "Right Stage" {
                        n148 = Unbundle By Name(w294) -> ("Stage X Axis (Volts/um)"=w290:dbl)
                        n149 = Unbundle By Name(w292) -> ("X Axis Voltage (I16)"=w289:i16)
                        n150 = Multiply(x=w293, y=w290) -> (x*y=w287:dbl)
                        n151 = call "Volts to I16.vi"("Voltage (V)"=w287) -> ("I16"=w286:i16)  [unwired: 13 in, 1 out]
                        n152 = Add(x=w289, y=w286) -> (x+y=w288:i16)
                        n153 = Bundle By Name(cluster=w292, "X Axis Voltage (I16)"=w288) -> (w291:T10)
                      }
                    }
                    n154 = call "Manual Controls Action Engine.vi"("Action"=enum16{"Read", "Write"}."Write", "Manual Controls In"=w248) -> ("Manual Controls Out"=w245:T10)  [unwired: 13 in]
                    n155 = call "FPGA-7842R-Control V1.vi"("Action"=FPGA-7842R-Reference."Stage Control", "Manual Controls"=w245, "Initialize"=TRUE) -> ()  [unwired: 11 in, 2 out]
                  }
                }
                n156 = Build Array(w236, w236) -> (w235:bool[])
                n157 = call "M686.vi"("Abort"=w238, "Axis"=w235, "Action"=StageStates."JOYSTICK", "VISA In"=w243) -> ("VISA Out"=w234:refnum<visa-resource-name>)  [unwired: 4 in, 3 out]
                n158 = call "M686.vi"("Abort"=w238, "Action"=StageStates."POSITION", "VISA In"=w234) -> ("Position Out"=w240:dbl[])  [unwired: 5 in, 3 out]
              }
            }
            n159 = Index Array(array=w123) -> (element #1=w121:dbl, element #2=w120:dbl)  [unwired: 2 in]
            n160 = property on="Y Position" class="DigNum (strict)"("Value"=w121) -> ()  [unwired: 2 in, 2 out]
            n161 = property on="Step Size (um)" class="Enum (strict)"("Value"=w120) -> ()  [unwired: 2 in, 2 out]
          }
          frame Enabled {
          }
        }
      }
      event Value Change {
        w318 = FALSE ("element")
        n162 = event-data() -> ()  [unwired: 1 in, 6 out]
        n163 = Unbundle By Name("Laser Controls") -> ("STED"=w324:bool, "640 nm"=w321:bool, "590 nm"=w322:bool, "485 nm"=w323:bool, "590 Power (V)"=w315:dbl, "STED Power (V)"=w314:dbl, "Manual Control"=w303:bool)
        n164 = call "LASERs_ Crl_AE.vi"("Action"=enum16{"READ", "WRITE"}."WRITE", "Detectors Parameters In"="Laser Controls") -> ()  [unwired: 9 in, 1 out]
        n165 = Build Array(w324, w321, w322, w323, w318, w318, w318, w318) -> (w320:bool[])
        n166 = local read "Live"() -> (w304:bool)
        n167 = Boolean Array To Number(Boolean array=w320) -> (number=w319:u32)
        n168 = To Unsigned Byte Integer(number=w319) -> (unsigned 8bit integer=w317:u8)
        n169 = Or(x=w304, y=w303) -> (x .or. y?=w302:bool)
        n170 = In Range and Coerce(upper limit=3.0, x=w315, lower limit=0.0) -> (coerced(x)=w309:dbl)  [unwired: 1 out]
        n171 = In Range and Coerce(upper limit=5.0, x=w314, lower limit=0.0) -> (coerced(x)=w308:dbl)  [unwired: 1 out]
        n172 = call "U8_To_U32.vi"("U8 IN"=w317) -> ("U32 OUT"=w316:u32)  [unwired: 13 in, 1 out]
        n173 = call "Volts to I16.vi"("Voltage (V)"=w309) -> ("I16"=w307:i16)  [unwired: 13 in, 1 out]
        n174 = call "Volts to I16.vi"("Voltage (V)"=w308) -> ("I16"=w306:i16)  [unwired: 13 in, 1 out]
        n175 = case shown="True" w302 {
          tunnel: "Laser Controls" -> [_ w330]
          frame False {
          }
          frame True {
            n176 = call "FPGA-7842R-Control V1.vi"("Action"=FPGA-7842R-Reference."Laser Control", "Laser Controls"=w330, "Initialize"=TRUE) -> ()  [unwired: 11 in, 2 out]
          }
        }
        n177 = call "Scan Parameters Action Engine.vi"("Action"=enum16{"Read", "Write"}."Read") -> ("Scan Parameters OUT"=w327:T11)  [unwired: 14 in]
        n178 = Bundle By Name(cluster=w327, "Laser_States _U32"=w316, "590_Voltage_I16"=w307, "775_AOM_Volt_I16"=w306) -> (w325:T11)
        n179 = call "Scan Parameters Action Engine.vi"("Action"=enum16{"Read", "Write"}."Write", "Scan Parameters IN"=w325) -> ()  [unwired: 13 in, 1 out]
      }
      event Value Change {
        n180 = event-data() -> ()  [unwired: 1 in, 6 out]
        n181 = call "Detectors Crl_AE.vi"("Action"=enum16{"READ", "WRITE"}."WRITE", "Detectors Parameters In"="Detectors") -> ()  [unwired: 9 in, 1 out]
      }
      event Value Change {
        n182 = event-data() -> ("OldVal"=w356:T9, "NewVal"=w349:T9)  [unwired: 1 in]
        n183 = Not Equal?(x=w356, y=w349) -> (x != y?=w355:T22)
        n184 = Unbundle By Name(w355) -> ("Scan Mode"=w354:bool, "Image Dimension (um)"=w336:bool[], "Image Format"=w344:bool, "Pixel Size (nm)"=w335:bool[])
        n185 = Or Array Elements(Boolean array=w335) -> (logical OR=w348:bool)
        n186 = case shown="True" w348 {
          tunnel: w349 -> [w370 w378]
          tunnel: [w370 w376] -> w347
          tunnel: w335 -> [_ w374]
          frame False {
          }
          frame True {
            n187 = Unbundle By Name(w378) -> ("Pixel Size (nm)"=w373:dbl[], "Image Format"=w382:u16)
            n188 = for {
              tunnel: w374 -> [w383] mode=indexing
              tunnel: w373 -> [w384] mode=indexing
              tunnel: [w384] -> w375
              stop <- w383 stop-if-true
            }
            n189 = Array Size(array=w373) -> (size(s)=w372:i32)
            n190 = To Double Precision Float(number=w382) -> (double precision float=w380:dbl)
            n191 = Initialize Array(w375, w372) -> (w371:dbl[])
            n192 = Multiply(x=w371, y=w380) -> (x*y=w381:dbl[])
            n193 = Multiply(x=w381, y=0.001) -> (x*y=w377:dbl[])
            n194 = Bundle By Name(cluster=w378, "Pixel Size (nm)"=w371, "Image Dimension (um)"=w377) -> (w376:T9)
          }
        }
        n195 = Or Array Elements(Boolean array=w336) -> (logical OR=w346:bool)
        n196 = Or(x=w346, y=w344) -> (x .or. y?=w345:bool)
        n197 = case shown="True" w354 {
          tunnel: w349 -> [_ w401]
          tunnel: w356 -> [_ w402]
          frame False {
          }
          frame True {
            n198 = control-ref of="Channel 1"() -> (w400:refnum<vi>)
            n199 = call "Select_Focus_Plane.vi"("NewVal"=w401, "OldVal"=w402, "IntensityGraph in"=w400) -> ()  [unwired: 9 in]
          }
        }
        n200 = case shown="True" w345 {
          tunnel: w347 -> [w385 w393]
          tunnel: [w385 w391] -> w339
          tunnel: w336 -> [_ w390]
          frame False {
          }
          frame True {
            n201 = Unbundle By Name(w393) -> ("Image Dimension (um)"=w387:dbl[], "Image Format"=w397:u16)
            n202 = for {
              tunnel: w390 -> [w398] mode=indexing
              tunnel: w387 -> [w399] mode=indexing
              tunnel: [w399] -> w389
              stop <- w398 stop-if-true
            }
            n203 = Array Size(array=w387) -> (size(s)=w386:i32)
            n204 = To Double Precision Float(number=w397) -> (double precision float=w395:dbl)
            n205 = Initialize Array(w389, w386) -> (w388:dbl[])
            n206 = Divide(x=w388, y=w395) -> (x/y=w396:dbl[])
            n207 = Multiply(x=w396, y=1000.0) -> (x*y=w392:dbl[])
            n208 = Bundle By Name(cluster=w393, "Image Dimension (um)"=w388, "Pixel Size (nm)"=w392) -> (w391:T9)
          }
        }
        n209 = Unbundle By Name(w339) -> ("Image Dimension (um)"=w357:dbl[], "Scan Type"=w362:enum16{"Sample Scanning", "Beam Scanning"})
        n210 = Equal?(x=w362, y=enum16{"Sample Scanning", "Beam Scanning"}."Beam Scanning") -> (x = y?=w340:bool)
        n211 = Index Array(array=w357, index=0) -> (element=w364:dbl)
        n212 = call "Res Mirror um to Volts.vi"("Image Size (um)"=w364) -> ("Voltage (V)"=w365:dbl)
        n213 = Select(t=15780.0, s=w340, f=100.0) -> (s? t:f=w341:dbl)
        n214 = In Range and Coerce(upper limit=5.0, x=w365, lower limit=0.0) -> (coerced(x)=w366:dbl)  [unwired: 1 out]
        n215 = Bundle By Name(cluster=w339, "Fast Axis Frequency (Hz)"=w341) -> (w338:T9)
        n216 = call "Volts to I16.vi"("Voltage (V)"=w366) -> ("I16"=w361:i16)  [unwired: 13 in, 1 out]
        n217 = call "Manual Controls Action Engine.vi"("Action"=enum16{"Read", "Write"}."Read") -> ("Manual Controls Out"=w352:T10)  [unwired: 14 in]
        n218 = Bundle By Name(cluster=w352, "Res Mirror Amp (I16)"=w361, "Res Mirror Mute"=w340) -> (w350:T10)
        n219 = call "Image Aquisition Param Ctrl_AE.vi"("Action"=enum16{"READ", "WRITE"}."WRITE", "Image Acquisition Parameters In"=w338) -> ()  [unwired: 9 in, 1 out]
        n220 = call "FPGA-7842R-Control V1.vi"("Action"=FPGA-7842R-Reference."Set Res Mirror", "Manual Controls"=w350, "Initialize"=TRUE) -> ()  [unwired: 11 in, 2 out]
        n221 = call "Manual Controls Action Engine.vi"("Action"=enum16{"Read", "Write"}."Write", "Manual Controls In"=w350) -> ()  [unwired: 13 in, 1 out]
      }
      event Value Change {
        n222 = event-data() -> ("CtlRef"=w407:refnum<vi>)  [unwired: 1 in, 2 out]
        n223 = property class="Bool"(reference=w407) -> ("Label.Text"=w406:string)  [unwired: 1 in, 2 out]
        n224 = call "Image Aquisition Param Ctrl_AE.vi"("Action"=enum16{"READ", "WRITE"}."READ") -> ("Image Acquisition Parameters Out"=w404:T9)  [unwired: 10 in]
        n225 = case shown="\"ZoomDown\"" w406 {
          tunnel: w404 -> [w410 w420 w476]
          tunnel: "Focus Control" -> [_ w419 w475]
          frame "SetZoom", Default {
            n226 = control-ref of="Channel 1"() -> (w409:refnum<vi>)
            n227 = call "Set_Focus_Plane.vi"("Image Acquisition Parameters Out"=w410, "IntensityGraph in"=w409) -> ()  [unwired: 10 in]
          }
          frame "ZoomUp" {
            n228 = Unbundle By Name(w419) -> ("ZoomStepI16"=w416:enum16{"Coarse", "Medium", "Fine"})
            n229 = Unbundle By Name(w420) -> ("Scan Type"=w418:enum16{"Sample Scanning", "Beam Scanning"}, "Scan Mode"=w417:enum16{"XY", "XZ", "YZ", "XYZ"})
            n230 = case shown="\"Medium\"" w416 {
              tunnel: [i16 500 i16 150 i16 50] -> w414
              frame "Coarse", Default {
              }
              frame "Medium" {
              }
              frame "Fine" {
              }
            }
            n231 = call "Manual Controls Action Engine.vi"("Action"=enum16{"Read", "Write"}."Read") -> ("Manual Controls Out"=w415:T10)  [unwired: 14 in]
            n232 = case shown="\"Beam Scanning\"" w418 {
              tunnel: w417 -> [w434 w460]
              tunnel: w415 -> [w433 w459]
              tunnel: w414 -> [w432 w458]
              tunnel: [w431 w455] -> w413
              frame "Sample Scanning", Default {
                n233 = case shown="\"YZ\"" w434 {
                  tunnel: w433 -> [w439 w444 w449 w454]
                  tunnel: w432 -> [w437 w442 w447 w452]
                  tunnel: [w436 w441 w446 w451] -> w431
                  tunnel: [w435 w440 w445 w450] -> w428
                  frame "XZ" {
                    n234 = Unbundle By Name(w439) -> ("Y Axis Voltage (I16)"=w438:i16)
                    n235 = Add(x=w438, y=w437) -> (x+y=w435:i16)
                    n236 = Bundle By Name(cluster=w439, "Y Axis Voltage (I16)"=w435) -> (w436:T10)
                  }
                  frame "YZ" {
                    n237 = Unbundle By Name(w444) -> ("X Axis Voltage (I16)"=w443:i16)
                    n238 = Add(x=w443, y=w442) -> (x+y=w440:i16)
                    n239 = Bundle By Name(cluster=w444, "X Axis Voltage (I16)"=w440) -> (w441:T10)
                  }
                  frame "XYZ" {
                    n240 = Unbundle By Name(w449) -> ("Z Axis Voltage (I16)"=w448:i16)
                    n241 = Add(x=w448, y=w447) -> (x+y=w445:i16)
                    n242 = Bundle By Name(cluster=w449, "Z Axis Voltage (I16)"=w445) -> (w446:T10)
                  }
                  frame "XY" {
                    n243 = Unbundle By Name(w454) -> ("Z Axis Voltage (I16)"=w453:i16)
                    n244 = Add(x=w453, y=w452) -> (x+y=w450:i16)
                    n245 = Bundle By Name(cluster=w454, "Z Axis Voltage (I16)"=w450) -> (w451:T10)
                  }
                }
                n246 = call "FPGA-7842R-Control V1.vi"("Action"=FPGA-7842R-Reference."Unused Axis I16", "Initialize"=TRUE, "Unused Axis Offset (I16)"=w428) -> ()  [unwired: 11 in, 2 out]
                n247 = call "Scan Parameters Action Engine.vi"("Action"=enum16{"Read", "Write"}."Read") -> ("Scan Parameters OUT"=w427:T11)  [unwired: 14 in]
                n248 = Bundle By Name(cluster=w427, "Unused_Axis_I16"=w428) -> (w426:T11)
                n249 = call "Scan Parameters Action Engine.vi"("Action"=enum16{"Read", "Write"}."Write", "Scan Parameters IN"=w426) -> ()  [unwired: 13 in, 1 out]
              }
              frame "Beam Scanning" {
                n250 = case shown="\"XY\", Default" w460 {
                  tunnel: w459 -> [w465]
                  tunnel: w458 -> [w463]
                  tunnel: [w462] -> w455
                  frame "XY", Default {
                    n251 = Unbundle By Name(w465) -> ("Z Axis Voltage (I16)"=w464:i16)
                    n252 = Add(x=w464, y=w463) -> (x+y=w461:i16)
                    n253 = Bundle By Name(cluster=w465, "Z Axis Voltage (I16)"=w461) -> (w462:T10)
                  }
                }
                n254 = call "FPGA-7842R-Control V1.vi"("Action"=FPGA-7842R-Reference."Stage Control", "Manual Controls"=w455, "Initialize"=TRUE) -> ()  [unwired: 11 in, 2 out]
              }
            }
            n255 = call "Manual Controls Action Engine.vi"("Action"=enum16{"Read", "Write"}."Write", "Manual Controls In"=w413) -> ()  [unwired: 13 in, 1 out]
          }
          frame "ZoomDown" {
            n256 = Unbundle By Name(w476) -> ("Scan Type"=w474:enum16{"Sample Scanning", "Beam Scanning"}, "Scan Mode"=w473:enum16{"XY", "XZ", "YZ", "XYZ"})
            n257 = Unbundle By Name(w475) -> ("ZoomStepI16"=w472:enum16{"Coarse", "Medium", "Fine"})
            n258 = case shown="\"Medium\"" w472 {
              tunnel: [i16 500 i16 150 i16 50] -> w468
              frame "Coarse", Default {
              }
              frame "Medium" {
              }
              frame "Fine" {
              }
            }
            n259 = call "Manual Controls Action Engine.vi"("Action"=enum16{"Read", "Write"}."Read") -> ("Manual Controls Out"=w470:T10)  [unwired: 14 in]
            n260 = Negate(x=w468) -> (-x=w466:i16)
            n261 = case shown="\"Sample Scanning\"" w474 {
              tunnel: w473 -> [w490 w516 _]
              tunnel: w470 -> [w489 w515 w522]
              tunnel: w466 -> [w488 w514 _]
              tunnel: [w487 w511 w522] -> w467
              frame "Sample Scanning" {
                n262 = case shown="\"XYZ\"" w490 {
                  tunnel: w489 -> [w495 w500 w505 w510]
                  tunnel: w488 -> [w493 w498 w503 w508]
                  tunnel: [w492 w497 w502 w507] -> w487
                  tunnel: [w491 w496 w501 w506] -> w480
                  frame "XZ" {
                    n263 = Unbundle By Name(w495) -> ("Y Axis Voltage (I16)"=w494:i16)
                    n264 = Add(x=w494, y=w493) -> (x+y=w491:i16)
                    n265 = Bundle By Name(cluster=w495, "Y Axis Voltage (I16)"=w491) -> (w492:T10)
                  }
                  frame "YZ" {
                    n266 = Unbundle By Name(w500) -> ("X Axis Voltage (I16)"=w499:i16)
                    n267 = Add(x=w499, y=w498) -> (x+y=w496:i16)
                    n268 = Bundle By Name(cluster=w500, "X Axis Voltage (I16)"=w496) -> (w497:T10)
                  }
                  frame "XYZ" {
                    n269 = Unbundle By Name(w505) -> ("Z Axis Voltage (I16)"=w504:i16)
                    n270 = Add(x=w504, y=w503) -> (x+y=w501:i16)
                    n271 = Bundle By Name(cluster=w505, "Z Axis Voltage (I16)"=w501) -> (w502:T10)
                  }
                  frame "XY" {
                    n272 = Unbundle By Name(w510) -> ("Z Axis Voltage (I16)"=w509:i16)
                    n273 = Add(x=w509, y=w508) -> (x+y=w506:i16)
                    n274 = Bundle By Name(cluster=w510, "Z Axis Voltage (I16)"=w506) -> (w507:T10)
                  }
                }
                n275 = call "FPGA-7842R-Control V1.vi"("Action"=FPGA-7842R-Reference."Unused Axis I16", "Initialize"=TRUE, "Unused Axis Offset (I16)"=w480) -> ()  [unwired: 11 in, 2 out]
                n276 = call "Scan Parameters Action Engine.vi"("Action"=enum16{"Read", "Write"}."Read") -> ("Scan Parameters OUT"=w483:T11)  [unwired: 14 in]
                n277 = Bundle By Name(cluster=w483, "Unused_Axis_I16"=w480) -> (w484:T11)
                n278 = call "Scan Parameters Action Engine.vi"("Action"=enum16{"Read", "Write"}."Write", "Scan Parameters IN"=w484) -> ()  [unwired: 13 in, 1 out]
              }
              frame "Beam Scanning" {
                n279 = case shown="\"XY\", Default" w516 {
                  tunnel: w515 -> [w521]
                  tunnel: w514 -> [w519]
                  tunnel: [w518] -> w511
                  tunnel: [w517] -> _
                  frame "XY", Default {
                    n280 = Unbundle By Name(w521) -> ("Z Axis Voltage (I16)"=w520:i16)
                    n281 = Add(x=w520, y=w519) -> (x+y=w517:i16)
                    n282 = Bundle By Name(cluster=w521, "Z Axis Voltage (I16)"=w517) -> (w518:T10)
                  }
                }
                n283 = call "FPGA-7842R-Control V1.vi"("Action"=FPGA-7842R-Reference."Stage Control", "Manual Controls"=w511, "Initialize"=TRUE) -> ()  [unwired: 11 in, 2 out]
              }
              frame Default {
              }
            }
            n284 = call "Manual Controls Action Engine.vi"("Action"=enum16{"Read", "Write"}."Write", "Manual Controls In"=w467) -> ()  [unwired: 13 in, 1 out]
          }
        }
      }
      event "Active Channel", "Colormap", "Graph Mode", "Cursor": Value Change {
        n285 = event-data() -> ("CtlRef"=w526:refnum<vi>)  [unwired: 1 in, 5 out]
        n286 = property class="Ctl"(reference=w526) -> ("Label.Text"=w525:string)  [unwired: 1 in, 2 out]
        n287 = call "Graph Ref AE.vi"("Action"=enum16{"READ", "WRITE"}."READ") -> ("Graph Ref Out"=w524:refnum<vi>[])  [unwired: 10 in]
        n288 = case shown="\"Cursor\"" w525 {
          tunnel: w524 -> [w531 w563 w589 w600]
          tunnel: "Active Channel" -> [w530 w562 w588 _]
          frame "Colormap", Default {
            n289 = To Long Integer(number=w530) -> (32bit integer=w529:i32)
            n290 = Index Array(array=w531, index=w529) -> (element=w533:refnum<vi>)
            n291 = property class="IntGraph (strict)"(reference=w533) -> (reference out=w535:refnum<vi>, "ZScale.Maximum"=w534:dbl)  [unwired: 1 in, 1 out]
            n292 = case shown="\"Green-White\"" "Colormap" {
              tunnel: [cluster{dbl, u32}[] [{0.0, 0}, {85.0, 16711680}, {108.0, 16729344}, {127.0, 16744192}, {132.0, 16747520}, {140.0, 16753920}, {157.0, 16766720}, {170.0, 16776960}, {245.0, 16777184}, {250.0, 16777200}, {255.0, 16777215}] ("Z Scale.Marker Values[]") cluster{dbl, u32}[] [{0.0, 0}, {255.0, 16777215}] ("Z Scale.Marker Values[]") cluster{dbl, u32}[] [{0.0, 0}, {255.0, 16711680}] ("Z Scale.Marker Values[]") cluster{dbl, u32}[] [{0.0, 0}, {255.0, 65280}] ("Z Scale.Marker Values[]") cluster{dbl, u32}[] [{0.0, 0}, {255.0, 255}] ("Z Scale.Marker Values[]") cluster{dbl, u32}[] [{0.0, 0}, {255.0, 65535}] ("Z Scale.Marker Values[]") cluster{dbl, u32}[] [{0.0, 0}, {255.0, 16711935}] ("Z Scale.Marker Values[]") cluster{dbl, u32}[] [{0.0, 0}, {255.0, 16776960}] ("Z Scale.Marker Values[]") cluster{dbl, u32}[] [{0.0, 0}, {170.0, 16711680}, {245.0, 16777184}, {250.0, 16777200}, {255.0, 16448250}] ("Z Scale.Marker Values[]") cluster{dbl, u32}[] [{0.0, 0}, {170.0, 65280}, {245.0, 16777184}, {250.0, 16777200}, {255.0, 16448250}] ("Z Scale.Marker Values[]") cluster{dbl, u32}[] [{0.0, 0}, {170.0, 255}, {245.0, 16777184}, {250.0, 16777200}, {255.0, 16448250}] ("Z Scale.Marker Values[]") cluster{dbl, u32}[] [{0.0, 0}, {1.0, 131072}, {2.0, 196608}, {3.0, 327680}, {4.0, 458752}, {5.0, 589824}, {6.0, 720896}, {7.0, 851971}, {8.0, 983043}, {9.0, 1114115}, {10.0, 1245187}, {11.0, 1376259}, {12.0, 1507331}, {13.0, 1638403}, {14.0, 1769475}, {15.0, 1769479}, {16.0, 2031623}, {17.0, 2162695}, {18.0, 2293767}, {19.0, 2424839}, {20.0, 2555911}, {21.0, 2686983}, {22.0, 2818055}, {23.0, 2949127}, {24.0, 3080203}, {25.0, 3211275}, {26.0, 3342347}, {27.0, 3473419}, {28.0, 3604491}, {29.0, 3735563}, {30.0, 3866635}, {31.0, 3867403}, {32.0, 4129547}, {33.0, 4260619}, {34.0, 4391691}, {35.0, 4522763}, {36.0, 4653839}, {37.0, 4784911}, {38.0, 4915983}, {39.0, 5178127}, {40.0, 5309199}, {41.0, 5440271}, {42.0, 5571343}, {43.0, 5702415}, {44.0, 5703439}, {45.0, 5965583}, {46.0, 6096655}, {47.0, 6227727}, {48.0, 6358799}, {49.0, 6489871}, {50.0, 6620943}, {51.0, 6752015}, {52.0, 6883087}, {53.0, 7015183}, {54.0, 7146255}, {55.0, 7277327}, {56.0, 7408399}, {57.0, 7539471}, {58.0, 7670543}, {59.0, 7801615}, {60.0, 8063759}, {61.0, 8194831}, {62.0, 8326927}, {63.0, 8457999}, {64.0, 8589075}, {65.0, 8720147}, {66.0, 8851219}, {67.0, 8982291}, {68.0, 9113363}, {69.0, 9114387}, {70.0, 9376531}, {71.0, 9507603}, {72.0, 9638675}, {73.0, 9769747}, {74.0, 9901843}, {75.0, 10032915}, {76.0, 10163987}, {77.0, 10229523}, {78.0, 10295059}, {79.0, 10427155}, {80.0, 10558227}, {81.0, 10689299}, {82.0, 10820371}, {83.0, 10886931}, {84.0, 10952467}, {85.0, 11083539}, {86.0, 11214611}, {87.0, 11215635}, {88.0, 11477779}, {89.0, 11543315}, {90.0, 11608851}, {91.0, 11740947}, {92.0, 11806483}, {93.0, 11872019}, {94.0, 12004115}, {95.0, 12135187}, {96.0, 12266259}, {97.0, 12267283}, {98.0, 12398355}, {99.0, 12529427}, {100.0, 12530451}, {101.0, 12595987}, {102.0, 12530451}, {103.0, 12793619}, {104.0, 12794131}, {105.0, 12794643}, {106.0, 13056787}, {107.0, 13057299}, {108.0, 13057811}, {109.0, 13188883}, {110.0, 13320979}, {111.0, 13386515}, {112.0, 13452563}, {113.0, 13584147}, {114.0, 13584659}, {115.0, 13585171}, {116.0, 13585683}, {117.0, 13717267}, {118.0, 13848339}, {119.0, 13849363}, {120.0, 13849875}, {121.0, 13850387}, {122.0, 13981459}, {123.0, 14113555}, {124.0, 14114067}, {125.0, 14114579}, {126.0, 14115091}, {127.0, 14246675}, {128.0, 14377747}, {129.0, 14378771}, {130.0, 14379283}, {131.0, 14379539}, {132.0, 14379795}, {133.0, 14380819}, {134.0, 14511891}, {135.0, 14643987}, {136.0, 14644503}, {137.0, 14645015}, {138.0, 14645527}, {139.0, 14646039}, {140.0, 14646551}, {141.0, 14778135}, {142.0, 14909207}, {143.0, 14910231}, {144.0, 14910747}, {145.0, 14911259}, {146.0, 14911771}, {147.0, 14912283}, {148.0, 14912797}, {149.0, 15044383}, {150.0, 15175455}, {151.0, 15175967}, {152.0, 15176479}, {153.0, 15176991}, {154.0, 15177507}, {155.0, 15178019}, {156.0, 15178531}, {157.0, 15310115}, {158.0, 15441701}, {159.0, 15441959}, {160.0, 15442215}, {161.0, 15442727}, {162.0, 15443243}, {163.0, 15443755}, {164.0, 15444269}, {165.0, 15444783}, {166.0, 15444783}, {167.0, 15576367}, {168.0, 15707953}, {169.0, 15708467}, {170.0, 15708979}, {171.0, 15708981}, {172.0, 15708983}, {173.0, 15710011}, {174.0, 15710523}, {175.0, 15711037}, {176.0, 15711039}, {177.0, 15711553}, {178.0, 15843139}, {179.0, 15974213}, {180.0, 15974215}, {181.0, 15974217}, {182.0, 15974219}, {183.0, 15975755}, {184.0, 15976271}, {185.0, 15976785}, {186.0, 15977299}, {187.0, 15977301}, {188.0, 15977815}, {189.0, 15978327}, {190.0, 15978331}, {191.0, 16109917}, {192.0, 16241503}, {193.0, 16241505}, {194.0, 16242019}, {195.0, 16242535}, {196.0, 16242537}, {197.0, 16242539}, {198.0, 16243563}, {199.0, 16243567}, {200.0, 16244081}, {201.0, 16244595}, {202.0, 16244599}, {203.0, 16244601}, {204.0, 16244603}, {205.0, 16245627}, {206.0, 16245631}, {207.0, 16245633}, {208.0, 16246147}, {209.0, 16246663}, {210.0, 16377735}, {211.0, 16508811}, {212.0, 16508815}, {213.0, 16509839}, {214.0, 16509843}, {215.0, 16509845}, {216.0, 16509847}, {217.0, 16510361}, {218.0, 16510875}, {219.0, 16510879}, {220.0, 16510881}, {221.0, 16510883}, {222.0, 16511399}, {223.0, 16511911}, {224.0, 16511915}, {225.0, 16511917}, {226.0, 16511919}, {227.0, 16511923}, {228.0, 16512437}, {229.0, 16512951}, {230.0, 16512955}, {231.0, 16512957}, {232.0, 16512959}, {233.0, 16512961}, {234.0, 16512963}, {235.0, 16512967}, {236.0, 16513481}, {237.0, 16513995}, {238.0, 16513999}, {239.0, 16514001}, {240.0, 16514003}, {241.0, 16514005}, {242.0, 16514007}, {243.0, 16514011}, {244.0, 16514013}, {245.0, 16514015}, {246.0, 16514019}, {247.0, 16514021}, {248.0, 16514023}, {249.0, 16514027}, {250.0, 16514029}, {251.0, 16514031}, {252.0, 16514035}, {253.0, 16514037}, {254.0, 16514039}, {255.0, 16514043}] ("Z Scale.Marker Values[]")] -> w537
              tunnel: [w538 w540 w542 w544 w546 w548 w550 w552 w554 w556 w558 w560] -> w536
              tunnel: w534 -> [w538 w540 w542 w544 w546 w548 w550 w552 w554 w556 w558 w560]
              frame "Fire", Default {
                # "Fire"
              }
              frame "Gray" {
                # "Grayscale"
              }
              frame "Red" {
                # "Red"
              }
              frame "Green" {
                # "Green"
              }
              frame "Blue" {
                # "Blue"
              }
              frame "Cyan" {
                # "Cyan"
              }
              frame "Magenta" {
                # "Magenta"
              }
              frame "Yellow" {
                # "Yellow"
              }
              frame "Red-White" {
                # "Red-White"
              }
              frame "Green-White" {
                # "Green-White"
              }
              frame "Blue-White" {
                # "Blue-White"
              }
              frame "Glow" {
              }
            }
            n293 = property class="IntGraph (strict)"(reference=w535, "ZScale.Maximum"=w536, "ZScale.MarkerVals[]"=w537) -> ()  [unwired: 1 in, 2 out]
          }
          frame "Graph Mode" {
            n294 = case shown="\"ZoomIn\"" "Graph Mode" {
              tunnel: w563 -> [w565 w569 w572 w575 w579]
              tunnel: w562 -> [_ _ _ _ w578]
              frame "FullChip" {
                n295 = for {
                  tunnel: w565 -> [w568] mode=indexing
                  n296 = property class="IntGraph (strict)"(reference=w568, "ActPaletteTool"=5 ("Palette:Active Tool"), "ZScale.ScaleFit"=u8 1 ("Z Scale.Scale Fit")) -> ()  [unwired: 1 in, 2 out]
                }
              }
              frame "ZoomIn" {
                n297 = for {
                  tunnel: w569 -> [w570] mode=indexing
                  n298 = property on="Property Node" class="IntGraph (strict)"(reference=w570, "ActPaletteTool"=6 ("Palette:Active Tool")) -> ()  [unwired: 1 in, 2 out]
                }
              }
              frame "ZoomOut" {
                n299 = for {
                  tunnel: w572 -> [w573] mode=indexing
                  n300 = property on="Property Node" class="IntGraph (strict)"(reference=w573, "ActPaletteTool"=7 ("Palette:Active Tool")) -> ()  [unwired: 1 in, 2 out]
                }
              }
              frame "Pan" {
                n301 = for {
                  tunnel: w575 -> [w576] mode=indexing
                  n302 = property on="Property Node" class="IntGraph (strict)"(reference=w576, "ActPaletteTool"=1 ("Palette:Active Tool")) -> ()  [unwired: 1 in, 2 out]
                }
              }
              frame "GetIntensity" {
                n303 = for {
                  tunnel: w579 -> [w586] mode=indexing
                  tunnel: w578 -> [w580]
                  i -> [w581]
                  n304 = property on="Property Node" class="IntGraph (strict)"(reference=w586, "ActPaletteTool"=0 ("Palette:Active Tool")) -> (reference out=w582:refnum<vi>)  [unwired: 1 in, 1 out]
                  n305 = To Long Integer(number=w580) -> (32bit integer=w585:i32)
                  n306 = Equal?(x=w585, y=w581) -> (x = y?=w584:bool)
                  n307 = property class="IntGraph (strict)"(reference=w582, "ZScale.Visible"=w584, "ZScale.Position"=T16 {"Left"=2275, "Top"=-325} ("Z Scale.Position")) -> ()  [unwired: 1 in, 2 out]
                }
              }
            }
          }
          frame "Active Channel" {
            n308 = for {
              tunnel: w589 -> [w594] mode=indexing
              tunnel: w588 -> [w593]
              i -> [w592]
              n309 = To Long Integer(number=w593) -> (32bit integer=w590:i32)
              n310 = Equal?(x=w590, y=w592) -> (x = y?=w591:bool)
              n311 = property class="IntGraph (strict)"(reference=w594, "ZScale.Visible"=w591, "ZScale.Position"=T16 {"Left"=2275, "Top"=-325} ("Z Scale.Position")) -> ()  [unwired: 1 in, 2 out]
            }
          }
          frame "Cursor" {
            w597 = 100.0 ("Cursor.Cursor Position:Cursor X")
            n312 = Index Array(array=w600, index=0) -> (element=w598:refnum<vi>)
            n313 = property class="IntGraph (strict)"(reference=w598, "Cursor.Visible"="Cursor", "Cursor.Cursor X"=w597, "Cursor.Cursor Y"=w597) -> ()  [unwired: 1 in, 2 out]
          }
        }
      }
      event Value Change {
        n314 = event-data() -> ("OldVal"=w613:T3, "NewVal"=w612:T3)  [unwired: 1 in, 4 out]
        n315 = property on="Graph Tools" class="Clust"() -> ("Controls[]"=w606:refnum<vi>[])  [unwired: 2 in, 2 out]
        n316 = Not Equal?(x=w613, y=w612) -> (x != y?=w611:T3)
        n317 = local read "Active Channel"() -> (w603:u16)
        n318 = Cluster To Array(cluster=w611) -> (array=w610:bool[])
        n319 = for {
          tunnel: w610 -> [w701] mode=indexing
          tunnel: w606 -> [w700] mode=indexing
          tunnel: [w700] -> w609
          stop <- w701 stop-if-true
        }
        n320 = To Long Integer(number=w603) -> (32bit integer=w607:i32)
        n321 = property class="Ctl"(reference=w609) -> (reference out=w602:refnum<vi>, "Label.Text"=w608:string)  [unwired: 1 in, 1 out]
        n322 = call "Graph Ref AE.vi"("Action"=enum16{"READ", "WRITE"}."READ") -> ("Graph Ref Out"=w604:refnum<vi>[])  [unwired: 10 in]
        n323 = case shown="\"Fit\"" w608 {
          tunnel: w604 -> [_ w614 w627 w651 w656 _]
          tunnel: w607 -> [_ _ _ w650 w655 _]
          tunnel: w602 -> [_ _ _ _ _ w666]
          frame "False", Default {
          }
          frame "Add Display" {
            w617 = u16 0 items=["Read", "Write"] ("Action")
            w621 = u16 1 items=["Read", "Write"] ("Action")
            n324 = call "Arange_Displays_V2.vi"("Action"=w617) -> ("Number of Channels OUT"=w618:i32)  [unwired: 14 in]
            n325 = Increment(x=w618) -> (x+1=w620:i32)
            n326 = call "Arange_Displays_V2.vi"("Display References"=w614, "Action"=w621, "Number of Channels"=w620, "Aspect Ratio (h/w)"=1.0) -> ("Number of Channels OUT"=w615:i32)  [unwired: 11 in]
            n327 = for {
              N: w615 -> [_]
              tunnel: w614 -> [w626] mode=indexing
              tunnel: [w622] -> w616 mode=indexing
              i -> [w625]
              n328 = property class="IntGraph (strict)"(reference=w626) -> ("Label.Text"=w624:string)  [unwired: 1 in, 2 out]
              n329 = To Unsigned Word Integer(number=w625) -> (unsigned 16bit integer=w623:u16)
              n330 = Bundle("Label.Text"=w624, w623) -> (w622:cluster{"Label.Text":string, u16})  [unwired: 1 in]
            }
            n331 = property on="Active Channel" class="Ring (strict)"("StringsAndValues[]"=w616) -> ()  [unwired: 2 in, 2 out]
          }
          frame "Remove Display" {
            w630 = u16 0 items=["Read", "Write"] ("Action")
            w634 = u16 1 items=["Read", "Write"] ("Action")
            n332 = call "Arange_Displays_V2.vi"("Action"=w630) -> ("Number of Channels OUT"=w631:i32)  [unwired: 14 in]
            n333 = Decrement(x=w631) -> (x-1=w633:i32)
            n334 = call "Arange_Displays_V2.vi"("Display References"=w627, "Action"=w634, "Number of Channels"=w633, "Aspect Ratio (h/w)"=1.0) -> ("Number of Channels OUT"=w628:i32)  [unwired: 11 in]
            n335 = for {
              N: w628 -> [_]
              tunnel: w627 -> [w639] mode=indexing
              tunnel: [w635] -> w629 mode=indexing
              i -> [w638]
              n336 = property class="IntGraph (strict)"(reference=w639) -> ("Label.Text"=w637:string)  [unwired: 1 in, 2 out]
              n337 = To Unsigned Word Integer(number=w638) -> (unsigned 16bit integer=w636:u16)
              n338 = Bundle("Label.Text"=w637, w636) -> (w635:cluster{"Label.Text":string, u16})  [unwired: 1 in]
            }
            n339 = property on="Active Channel" class="Ring (strict)"("StringsAndValues[]"=w629) -> ()  [unwired: 2 in, 2 out]
          }
          frame "Load File" {
            w641 = u16 1 items=["Get Image", "Load and Read File"] ("Action")
            n340 = Index Array(array=w651, index=w650) -> (element=w640:refnum<vi>)
            n341 = call "OpenDBL.vi"("Action"=w641) -> ("Image"=w642:sgl[], "Dimensions (Z, Y, X, t)"=w643:i32[])  [unwired: 12 in, 1 out]
            n342 = Index Array(array=w643, index #1=1 ("index"), index #2=2 ("index")) -> (element #1=w646:i32, element #2=w647:i32)
            n343 = Reverse 1D Array(array=w642) -> (reversed array=w648:sgl[])
            n344 = Reshape Array(w648, w646, w647) -> (w649:sgl[][])
            n345 = property class="IntGraph (strict)"(reference=w640, "Value"=w649) -> ()  [unwired: 1 in, 2 out]
          }
          frame "Fit" {
            n346 = Index Array(array=w656, index=w655) -> (element=w654:refnum<vi>)
            n347 = local read "Image Acquisition Parameters"() -> (w653:T9)
            n348 = property class="IntGraph (strict)"(reference=w654) -> ("Value"=w662:sgl[][])  [unwired: 1 in, 2 out]
            n349 = vi-ref "QuickProfile_V3.vi"() -> (w657:refnum<vi>)
            n350 = property class="VI Interface Type 0"(reference=w657) -> ("Path"=w660:path)  [unwired: 1 in, 2 out]
            n351 = Unbundle By Name(w653) -> ("Pixel Size (nm)"=w652:dbl[])
            n352 = Index Array(array=w652, index=0) -> (element=w664:dbl)
            n353 = Open VI Reference(type specifier VI Refnum (for type only)=w657, vi path=w660, options=128) -> (vi reference=w658:refnum<vi>)  [unwired: 3 in, 1 out]
            n354 = call-by-ref "Start Asynchronous Call"(reference=w658, "Image IN"=w662, "Pixel Size (nm)"=w664) -> (reference out=w661:refnum<vi>)  [unwired: 15 in, 1 out]
            n355 = Close Reference(reference=w661) -> ()  [unwired: 1 in, 1 out]
          }
          frame "Single Screen" {
            n356 = property class="Ctl"(reference=w666) -> ("Value"=w665:variant)  [unwired: 1 in, 2 out]
            n357 = property class="App"() -> ("Disp.AllMonitors"=w670:T23)  [unwired: 2 in, 2 out]
            n358 = Variant To Data(type=FALSE, Variant=w665) -> (data=w667:bool)  [unwired: 1 in, 1 out]
            n359 = control-ref of="This VI"() -> (w669:refnum<vi>)
            n360 = case shown="True" w667 {
              tunnel: w670 -> [w674 w689]
              tunnel: T17 {"Left"=0, "Top"=0, "Right"=0, "Bottom"=0} ("FP Window Bounds 2") -> [w673 w688]
              tunnel: w669 -> [w672 w687]
              frame False {
                w683 = i16 0
                n361 = Index Array(array=w674, index #1=1 ("index"), index #2=0 ("index")) -> (element #1=w677:T24, element #2=w678:T24)
                n362 = Unbundle By Name(w678) -> ("Bounds.Left"=w680:i16, "Bounds.Bottom"=w681:i16, "Bounds.Top"=w682:i16)
                n363 = Unbundle By Name(w677) -> ("Bounds.Right"=w679:i16)
                n364 = Subtract(x=w679, y=w680) -> (x-y=w684:i16)
                n365 = Subtract(x=w681, y=w682) -> (x-y=w685:i16)
                n366 = Bundle By Name(cluster=w673, "Left"=w683, "Top"=w683, "Right"=w684, "Bottom"=w685) -> (w686:T17)
                n367 = property class="VI"(reference=w672, "Front Panel.WinBounds"=w686) -> ()  [unwired: 1 in, 2 out]
              }
              frame True {
                w692 = i16 0
                n368 = Index Array(array=w689, index=0) -> (element=w696:T24)
                n369 = Unbundle By Name(w696) -> ("Bounds.Right"=w697:i16, "Bounds.Bottom"=w694:i16, "Bounds.Top"=w693:i16)
                n370 = Subtract(x=w694, y=w693) -> (x-y=w691:i16)
                n371 = Bundle By Name(cluster=w688, "Left"=w692, "Top"=w692, "Right"=w697, "Bottom"=w691) -> (w690:T17)
                n372 = property class="VI"(reference=w687, "Front Panel.WinBounds"=w690) -> (reference out=w699:refnum<vi>)  [unwired: 1 in, 1 out]
                n373 = property class="VI"(reference=w699, "FP.State"=T18."Maximized" ("Front Panel Window:State")) -> ()  [unwired: 1 in, 2 out]
              }
            }
          }
        }
      }
      event "SLM", "Timing", "DM", "Pixelfly": Value Change {
        n374 = event-data() -> ("CtlRef"=w705:refnum<vi>, "NewVal"=w703:bool)  [unwired: 1 in, 4 out]
        n375 = property class="Bool (strict)"(reference=w705) -> ("Label.Text"=w704:string)  [unwired: 1 in, 2 out]
        n376 = case shown="\"SLM\"" w704 {
          tunnel: w703 -> [_ w706 w723 w739 w753]
          frame "False", Default {
          }
          frame "SLM" {
            n377 = case shown="True" w706 {
              frame False {
                n378 = call "SLM AE.vi"("Action"=enum16{"READ", "WRITE"}."READ") -> ("SLM Ref Out"=w713:refnum<vi>)  [unwired: 10 in]
                n379 = To Variant(anything=TRUE) -> (Variant=w712:variant)
                n380 = invoke class="VI" method="Ctrl Val.Set"(reference=w713, "Control Name"="Exit", "Value"=w712) -> (reference out=w709:refnum<vi>, error out=w708:errorcluster)  [unwired: 2 in, 3 out]
                n381 = disable-structure shown="Disabled" {
                  disable-tunnel: w708 -> [w716 w717]
                  disable-tunnel: [w715 w717] -> w707
                  frame Disabled {
                    n382 = invoke on="Hamamatsu LCOS" class="SubPnl" method="Remove VI"(error in=w716) -> (error out=w715:errorcluster)  [unwired: 2 in, 2 out]
                  }
                  frame Enabled {
                  }
                }
                n383 = Close Reference(reference=w709, error in (no error)=w707) -> ()  [unwired: 1 out]
              }
              frame True {
                n384 = Open VI Reference(vi path=path "C:/Users/ED STED/Documents/Test Control Software/Host VIs/SLM/SLM Control.vi") -> (vi reference=w721:refnum<vi>)  [unwired: 5 in, 1 out]
                n385 = invoke class="VI" method="Run VI"(reference=w721, "Wait until done"=FALSE ("Wait Until Done")) -> (reference out=w718:refnum<vi>)  [unwired: 3 in, 4 out]
                n386 = invoke on="Hamamatsu LCOS" class="SubPanel" method="Insert VI"("VI Ref"=w718) -> ()  [unwired: 3 in, 4 out]
                n387 = call "SLM AE.vi"("Action"=enum16{"READ", "WRITE"}."WRITE", "SLM Ref In"=w718) -> ()  [unwired: 9 in, 1 out]
              }
            }
          }
          frame "DM" {
            n388 = case shown="False" w723 {
              frame False {
                n389 = call "DM_Ref_AE.vi"("Action"=enum16{"READ", "WRITE"}."READ") -> ("DM Ref Out"=w730:refnum<vi>)  [unwired: 10 in]
                n390 = To Variant(anything=TRUE) -> (Variant=w729:variant)
                n391 = invoke class="VI" method="Ctrl Val.Set"(reference=w730, "Control Name"="Exit", "Value"=w729) -> (reference out=w726:refnum<vi>, error out=w725:errorcluster)  [unwired: 2 in, 3 out]
                n392 = disable-structure shown="Disabled" {
                  disable-tunnel: w725 -> [w733 _]
                  disable-tunnel: [w732 _] -> w724
                  frame Disabled {
                    n393 = invoke on="Hamamatsu LCOS" class="SubPnl" method="Remove VI"(error in=w733) -> (error out=w732:errorcluster)  [unwired: 2 in, 2 out]
                  }
                  frame Enabled {
                  }
                }
                n394 = Close Reference(reference=w726, error in (no error)=w724) -> ()  [unwired: 1 out]
              }
              frame True {
                n395 = Open VI Reference(vi path=path "C:/Users/STED/Desktop/Cambridge STED Control Software/Host VIs/DM/DM_Control_STED.vi") -> (vi reference=w737:refnum<vi>)  [unwired: 5 in, 1 out]
                n396 = invoke class="VI" method="Run VI"(reference=w737, "Wait until done"=FALSE ("Wait Until Done")) -> (reference out=w734:refnum<vi>)  [unwired: 3 in, 4 out]
                n397 = invoke on="BM Multi" class="SubPanel" method="Insert VI"("VI Ref"=w734) -> ()  [unwired: 3 in, 4 out]
                n398 = call "DM_Ref_AE.vi"("Action"=enum16{"READ", "WRITE"}."WRITE", "DM Ref In"=w734) -> ()  [unwired: 9 in, 1 out]
              }
            }
          }
          frame "Timing" {
            n399 = case shown="True" w739 {
              frame False {
                n400 = call "GateDelay AE.vi"("Action"=enum16{"READ", "WRITE"}."READ") -> ("Gate Delay Ref Out"=w746:refnum<vi>)  [unwired: 10 in]
                n401 = To Variant(anything=TRUE) -> (Variant=w745:variant)
                n402 = invoke class="VI" method="Ctrl Val.Set"(reference=w746, "Control Name"="Exit", "Value"=w745) -> (reference out=w741:refnum<vi>, error out=w742:errorcluster)  [unwired: 2 in, 3 out]
                n403 = invoke on="Timing" class="SubPnl" method="Remove VI"(error in=w742) -> (error out=w740:errorcluster)  [unwired: 2 in, 2 out]
                n404 = Close Reference(reference=w741, error in (no error)=w740) -> ()  [unwired: 1 out]
              }
              frame True {
                n405 = Open VI Reference(vi path=path "C:/Users/STED/Documents/STED VIs/Gate Delay Board/DelayBoardSTED.vi") -> (vi reference=w751:refnum<vi>)  [unwired: 5 in, 1 out]
                n406 = invoke class="VI" method="Run VI"(reference=w751, "Wait until done"=FALSE ("Wait Until Done")) -> (reference out=w748:refnum<vi>)  [unwired: 3 in, 4 out]
                n407 = invoke on="Timing" class="SubPanel" method="Insert VI"("VI Ref"=w748) -> ()  [unwired: 3 in, 4 out]
                n408 = call "GateDelay AE.vi"("Action"=enum16{"READ", "WRITE"}."WRITE", "Gate Delay Ref In"=w748) -> ()  [unwired: 9 in, 1 out]
              }
            }
          }
          frame "Pixelfly" {
            n409 = case shown="False" w753 {
              frame False {
                n410 = call "Pixelfly AE.vi"("Action"=enum16{"READ", "WRITE"}."READ") -> ("Gate Delay Ref Out"=w760:refnum<vi>)  [unwired: 10 in]
                n411 = To Variant(anything=TRUE) -> (Variant=w759:variant)
                n412 = invoke class="VI" method="Ctrl Val.Set"(reference=w760, "Control Name"="Exit", "Value"=w759) -> (reference out=w756:refnum<vi>, error out=w755:errorcluster)  [unwired: 2 in, 3 out]
                n413 = invoke on="Pixelfly" class="SubPnl" method="Remove VI"(error in=w755) -> (error out=w754:errorcluster)  [unwired: 2 in, 2 out]
                n414 = Close Reference(reference=w756, error in (no error)=w754) -> ()  [unwired: 1 out]
              }
              frame True {
                n415 = Open VI Reference(vi path=path "C:/Users/STED/Desktop/Cambridge STED Control Software/Host VIs/PCO_Pixelfly/PCO_Record.vi") -> (vi reference=w765:refnum<vi>)  [unwired: 5 in, 1 out]
                n416 = invoke class="VI" method="Run VI"(reference=w765, "Wait until done"=FALSE ("Wait Until Done")) -> (reference out=w762:refnum<vi>)  [unwired: 3 in, 4 out]
                n417 = invoke on="Pixelfly" class="SubPanel" method="Insert VI"("VI Ref"=w762) -> ()  [unwired: 3 in, 4 out]
                n418 = call "Pixelfly AE.vi"("Action"=enum16{"READ", "WRITE"}."WRITE", "Gate Delay Ref In"=w762) -> ()  [unwired: 9 in, 1 out]
              }
            }
          }
        }
      }
    }
  }
  n419 = while {
    shift-right: [w776] -> _
    shift-left: "Idle" -> [w777]
    tunnel: w26 -> [w773]
    shift-right: [w771] -> _
    shift-left: w23 -> [w772]
    stop <- w775 stop-if-true
    n420 = call "Image Aquisition Param Ctrl_AE.vi"("Action"=enum16{"READ", "WRITE"}."READ") -> ("Image Acquisition Parameters Out"=w770:T9)  [unwired: 10 in]
    n421 = call "Detectors Crl_AE.vi"("Action"=enum16{"READ", "WRITE"}."READ") -> ("Detectors Parameters Out"=w768:T7)  [unwired: 10 in]
    n422 = case shown="\"Stop Waveforms\"" w777 {
      selector: w777 -> [_ _ _ w809 _ _ _ _ _ _]
      tunnel: ["Exit" w786 "Idle" ("name (unnamed)") "Arange Displays" ("name (unnamed)") "Start FPGA Acquisition" ("name (unnamed)") "Display" ("name (unnamed)") "Close Images" ("name (unnamed)") "Idle" "Stop Waveforms" ("name (unnamed)") "Start Waveforms" ("name (unnamed)")] -> w776
      tunnel: [TRUE w788 w795 w817 w837 w858 w901 w934 w939 w945] -> w775
      tunnel: FALSE -> [_ w788 w795 w817 w837 w858 w901 w934 w939 w945]
      tunnel: w773 -> [_ w787 _ _ _ _ _ _ _ _]
      tunnel: w772 -> [w782 w785 w796 w815 w834 w856 w899 w932 w940 w946]
      tunnel: [w781 w785 w796 w815 w834 w852 w899 w931 w940 w946] -> w771
      tunnel: w770 -> [_ _ _ w808 _ w851 _ _ _ w943]
      tunnel: w768 -> [_ _ _ w807 _ _ _ _ _ w941]
      frame "Exit" {
        n423 = call "Graph Ref AE.vi"("Action"=enum16{"READ", "WRITE"}."READ") -> ("Graph Ref Out"=w779:refnum<vi>[])  [unwired: 10 in]
        n424 = call "FPGA-7842R-Control V1.vi"("Action"=FPGA-7842R-Reference."Close FPGA", "Initialize"=w782) -> ("Initalized"=w781:bool)  [unwired: 12 in, 1 out]
        n425 = Close Reference(reference=w779) -> ()  [unwired: 1 in, 1 out]
      }
      frame "Idle", Default {
        n426 = Dequeue Element(queue=w787, timeout in ms (-1)=-1) -> (element=w786:string)  [unwired: 1 in, 3 out]
      }
      frame "Close Images" {
        w791 = u16 0 items=["Read", "Write"] ("Mode")
        w792 = u16 0 items=["Write", "Read"] ("Mode")
        n427 = call "File Action V1.vi"("Mode"=w791) -> ("Files Open"=w790:bool)  [unwired: 12 in, 2 out]
        n428 = call "Image_Actions_V1.vi"("Mode"=w792, "Action"="Trash Images") -> ()  [unwired: 12 in, 2 out]
        n429 = case shown="True" w790 {
          frame False {
          }
          frame True {
            w798 = u16 1 items=["Read", "Write"] ("Mode")
            n430 = call "File Action V1.vi"("Action"="Close Files", "Mode"=w798) -> ()  [unwired: 11 in, 3 out]
          }
        }
      }
      frame "Capture", "Live" {
        w813 = u16 0 items=["Write", "Read"] ("Mode")
        n431 = Cluster To Array(cluster=w807) -> (array=w805:bool[])
        n432 = Index Array(array=w805, index=4) -> (element=w802:bool)
        n433 = Boolean To (0,1)(Boolean=w805) -> (0, 1=w806:i16[])
        n434 = Add Array Elements(numeric array=w806) -> (sum=w803:i16)
        n435 = To Long Integer(number=w803) -> (32bit integer=w800:i32)
        n436 = Unbundle By Name(w808) -> ("Image Format"=w810:u16)
        n437 = Select(t=1, s=w802, f=w800) -> (s? t:f=w799:i32)
        n438 = case shown="\"Capture\"" w809 {
          tunnel: w808 -> [_ w819]
          tunnel: w799 -> [_ w818]
          frame Default {
          }
          frame "Capture" {
            w822 = u16 1 items=["Read", "Write"] ("Mode")
            n439 = call "File Action V1.vi"("Action"="Open Files", "Mode"=w822, "Image Acquisition Parameters"=w819, "File Path IN"="Save File Path", "Number of Channels"=w818) -> ("File Path OUT"=w820:path)  [unwired: 8 in, 2 out]
            n440 = local write "Save File Path"(w820) -> ()
          }
        }
        n441 = To Long Integer(number=w810) -> (32bit integer=w812:i32)
        n442 = Bundle(w812, w812) -> (w811:cluster{i32, i32})  [unwired: 1 in]
        n443 = call "Image_Actions_V1.vi"("Image Size (Pixels)"=w811, "Mode"=w813, "Number of Channels"=w799, "Action"="Create Images") -> ()  [unwired: 10 in, 2 out]
      }
      frame "Arange Displays" {
        w832 = u16 1 items=["Write", "Read"] ("Mode")
        w835 = u16 1 items=["Read", "Write"] ("Action")
        n444 = call "Graph Ref AE.vi"("Action"=enum16{"READ", "WRITE"}."READ") -> ("Graph Ref Out"=w827:refnum<vi>[])  [unwired: 10 in]
        n445 = call "Image_Actions_V1.vi"("Mode"=w832) -> ("Image REFs OUT"=w833:T25[])  [unwired: 13 in, 1 out]
        n446 = Array Size(array=w833) -> (size(s)=w831:i32)
        n447 = call "Arange_Displays_V2.vi"("Display References"=w827, "Action"=w835, "Number of Channels"=w831, "Aspect Ratio (h/w)"=1.0) -> ("Number of Channels OUT"=w828:i32)  [unwired: 11 in]
        n448 = for {
          N: w828 -> [_]
          tunnel: w827 -> [w839] mode=indexing
          tunnel: [w842] -> w829 mode=indexing
          i -> [w840]
          n449 = property class="IntGraph (strict)"(reference=w839) -> ("Label.Text"=w844:string)  [unwired: 1 in, 2 out]
          n450 = Equal To 0?(x=w840) -> (x = 0?=w841:bool)
          n451 = case shown="True" w841 {
            tunnel: w839 -> [_ w845]
            frame False {
            }
            frame True {
              n452 = property class="IntGraph (strict)"(reference=w845, "ZScale.Visible"=TRUE ("Z Scale.Visible"), "ZScale.Position"=T16 {"Left"=2275, "Top"=-325} ("Z Scale.Position")) -> ()  [unwired: 1 in, 2 out]
            }
          }
          n453 = To Unsigned Word Integer(number=w840) -> (unsigned 16bit integer=w843:u16)
          n454 = Bundle("Label.Text"=w844, w843) -> (w842:cluster{"Label.Text":string, u16})  [unwired: 1 in]
        }
        n455 = property on="Active Channel" class="Ring (strict)"("StringsAndValues[]"=w829) -> (error out=w826:errorcluster)  [unwired: 2 in, 1 out]
        n456 = local write "Graph Mode"(T1."GetIntensity" ("Graph Mode")) -> ()
        n457 = property on="Active Channel" class="Ring (strict)"(error in=w826, "Value"=u16 0) -> ()  [unwired: 1 in, 2 out]
      }
      frame "Start Waveforms" {
        n458 = call "Initialize Waveforms V4.vi"("Image Acquisition Parameters"=w851) -> ("Waveform Data to FPGA"=w857:T26)  [unwired: 14 in]
        n459 = Unbundle By Name(w851) -> ("Scan Type"=w850:enum16{"Sample Scanning", "Beam Scanning"})
        n460 = call "FPGA-7842R-Control V1.vi"("Waveform Data"=w857, "Action"=FPGA-7842R-Reference."Start Waveforms", "Image Acquisition Parameters"=w851, "Initialize"=w856) -> ("Initalized"=w853:bool)  [unwired: 10 in, 1 out]
        n461 = Equal?(x=w850, y=enum16{"Sample Scanning", "Beam Scanning"}."Sample Scanning" ("Scan Type")) -> (x = y?=w848:bool)
        n462 = case shown="True" w848 {
          tunnel: w853 -> [w859 w864]
          tunnel: [w859 w863] -> w852
          frame False {
          }
          frame True {
            n463 = call "Scan Parameters Action Engine.vi"("Action"=enum16{"Read", "Write"}."Read") -> ("Scan Parameters OUT"=w861:T11)  [unwired: 14 in]
            n464 = Unbundle By Name(w861) -> ("Unused_Axis_I16"=w860:i16)
            n465 = call "FPGA-7842R-Control V1.vi"("Action"=FPGA-7842R-Reference."Unused Axis I16", "Initialize"=w864, "Unused Axis Offset (I16)"=w860) -> ("Initalized"=w863:bool)  [unwired: 11 in, 1 out]
          }
        }
      }
      frame "Display" {
        w893 = u16 1 items=["Write", "Read"] ("Mode")
        n466 = call "Image_Actions_V1.vi"("Mode"=w893) -> ("Image REFs OUT"=w895:T25[])  [unwired: 13 in, 1 out]
        n467 = Array Size(array=w895) -> (size(s)=w891:i32)
        n468 = Decrement(x=w891) -> (x-1=w890:i32)
        n469 = for {
          N: 6 -> [_]
          tunnel: w890 -> [w929]
          tunnel: [w927] -> w894 mode=indexing
          i -> [w928]
          n470 = Greater Or Equal?(x=w929, y=w928) -> (x >= y?=w927:bool)
        }
        n471 = Obtain Notifier(name (unnamed)="Running", notification data type=FALSE) -> (notifier out=w898:refnum<notifier>)  [unwired: 2 in, 2 out]
        n472 = Index Array(array=w894, index #1=1 ("index"), index #2=2 ("index"), index #3=3 ("index"), index #4=4 ("index"), index #5=5 ("index")) -> (element #1=w879:bool, element #2=w878:bool, element #3=w877:bool, element #4=w876:bool, element #5=w875:bool)
        n473 = Index Array(array=w895, index #1=0 ("index"), index #2=1 ("index"), index #3=2 ("index"), index #4=3 ("index"), index #5=4 ("index"), index #6=5 ("index")) -> (element #1=w874:T25, element #2=w873:T25, element #3=w872:T25, element #4=w871:T25, element #5=w870:T25, element #6=w869:T25)
        n474 = while {
          tunnel: w879 -> [w916]
          tunnel: w878 -> [w915]
          tunnel: w877 -> [w911]
          tunnel: w876 -> [w908]
          tunnel: w875 -> [w907]
          tunnel: w874 -> [w914]
          tunnel: w873 -> [w913]
          tunnel: w872 -> [w912]
          tunnel: w871 -> [w910]
          tunnel: w870 -> [w906]
          tunnel: w869 -> [w909]
          shift-right: [w902] -> w867
          shift-left: w898 -> [w902]
          stop <- w903 stop-if-true
          n475 = Get Notifier Status(notifier=w902) -> (current notification=w903:bool)  [unwired: 1 in, 4 out]
          n476 = case shown="False" w916 {
            tunnel: w913 -> [_ w926]
            frame False {
            }
            frame True {
              n477 = call "IMAQ ImageToArray"("Image"=w926) -> ("Image Pixels (Float)"=→"Channel 2":sgl[][])  [unwired: 3 in, 4 out]
            }
          }
          n478 = case shown="False" w915 {
            tunnel: w912 -> [_ w924]
            frame False {
            }
            frame True {
              n479 = call "IMAQ ImageToArray"("Image"=w924) -> ("Image Pixels (Float)"=→"Channel 3":sgl[][])  [unwired: 3 in, 4 out]
            }
          }
          n480 = call "IMAQ ImageToArray"("Image"=w914) -> ("Image Pixels (Float)"=→"Channel 1":sgl[][])  [unwired: 3 in, 4 out]
          n481 = case shown="False" w911 {
            tunnel: w910 -> [_ w922]
            frame False {
            }
            frame True {
              n482 = call "IMAQ ImageToArray"("Image"=w922) -> ("Image Pixels (Float)"=→"Channel 4":sgl[][])  [unwired: 3 in, 4 out]
            }
          }
          n483 = case shown="False" w908 {
            tunnel: w906 -> [_ w920]
            frame False {
            }
            frame True {
              n484 = call "IMAQ ImageToArray"("Image"=w920) -> ("Image Pixels (Float)"=→"Channel 5":sgl[][])  [unwired: 3 in, 4 out]
            }
          }
          n485 = case shown="False" w907 {
            tunnel: w909 -> [_ w918]
            frame False {
            }
            frame True {
              n486 = call "IMAQ ImageToArray"("Image"=w918) -> ("Image Pixels (Float)"=→"Channel 6":sgl[][])  [unwired: 3 in, 4 out]
            }
          }
          n487 = Wait (ms)(milliseconds to wait=u32 100) -> ()  [unwired: 1 out]
        }
        n488 = Release Notifier(notifier=w867, force destroy? (F)=FALSE) -> ()  [unwired: 1 in, 3 out]
      }
      frame "Stop Waveforms" {
        n489 = call "FPGA-7842R-Control V1.vi"("Action"=FPGA-7842R-Reference."Stop Waveforms", "Initialize"=w932) -> ("Initalized"=w931:bool)  [unwired: 12 in, 1 out]
      }
      frame "Stop Acquisition" {
        n490 = call "FPGA-7842R-Control V1.vi"("Action"=FPGA-7842R-Reference."Laser Control", "Laser Controls"=T8 {"STED Power (V)"=0.0, "590 Power (V)"=0.0, "STED"=FALSE, "640 nm"=FALSE, "590 nm"=FALSE, "485 nm"=FALSE, "Manual Control"=FALSE} ("Laser Controls 2"), "Initialize"=TRUE) -> ()  [unwired: 11 in, 2 out]
      }
      frame "Start FPGA Acquisition" {
        n491 = Unbundle By Name(w943) -> ("Scan Type"=w942:enum16{"Sample Scanning", "Beam Scanning"})
        n492 = case shown="\"Beam Scanning\"" w942 {
          tunnel: w943 -> [w948 w957]
          tunnel: w941 -> [w947 w958]
          frame "Sample Scanning", Default {
            n493 = disable-structure shown="Disabled" {
              disable-tunnel: w948 -> [w950 _]
              disable-tunnel: w947 -> [w949 _]
              frame Disabled {
                n494 = vi-ref "FPGA Sample Scanning V1.vi"() -> (w953:refnum<vi>)
                n495 = property class="VI Interface Type 1"(reference=w953) -> ("Path"=w951:path)  [unwired: 1 in, 2 out]
                n496 = Open VI Reference(type specifier VI Refnum (for type only)=w953, vi path=w951, options=128) -> (vi reference=w954:refnum<vi>)  [unwired: 3 in, 1 out]
                n497 = call-by-ref "Start Asynchronous Call"(reference=w954, "Detectors"=w949, "Image Acquisition Parameters"=w950) -> (reference out=w955:refnum<vi>)  [unwired: 2 in, 1 out]
                n498 = Close Reference(reference=w955) -> ()  [unwired: 1 in, 1 out]
              }
              frame Enabled {
              }
            }
          }
          frame "Beam Scanning" {
            n499 = vi-ref "FPGA Beam Scanning V1.vi"() -> (w956:refnum<vi>)
            n500 = property class="VI Interface Type 1"(reference=w956) -> ("Path"=w960:path)  [unwired: 1 in, 2 out]
            n501 = Open VI Reference(type specifier VI Refnum (for type only)=w956, vi path=w960, options=128) -> (vi reference=w959:refnum<vi>)  [unwired: 3 in, 1 out]
            n502 = call-by-ref "Start Asynchronous Call"(reference=w959, "Detectors"=w958, "Image Acquisition Parameters"=w957) -> (reference out=w962:refnum<vi>)  [unwired: 2 in, 1 out]
            n503 = Close Reference(reference=w962) -> ()  [unwired: 1 in, 1 out]
          }
        }
      }
    }
  }
